vi "Netway Cal UI.vi"(11 "Calling VI Ref":refnum<vi>) -> ()   [LabVIEW 2013]
uses:
  Netway Driver/Type Defs/Communication Function Type Def.ctl
  <vilib>/Utility/miscctls.llb/LVRowAndColumnTypeDef.ctl
  <vilib>/Analysis/NI_AALPro.lvlib
  Type Defs/Target Cluster Type Def.ctl
  Type Defs/Setpoint Cluster Type Def.ctl
  Type Defs/Targets Type Def (Netway).ctl
  <vilib>/Utility/config.llb/NI_LVConfig.lvlib
  <userlib>/_OpenG.lib/array/array.llb/Remove Duplicates from 1D Array (DBL)__ogtk.vi
  Type Defs/Units Type Def (Netway).ctl
  Type Defs/Input or Output Type Def.ctl
  Type Defs/Channel Type Def (Netway).ctl
  <userlib>/_OpenG.lib/array/array.llb/Filter 1D Array (DBL)__ogtk.vi
panel:
  in  "Output Value Tab":enum32{"Page 1", "Page 2"}(tab)
  in  "OK Output":bool
  in  "Cancel Output":bool
  in  "Output Reading":dbl
  in  "Load Indicator Tab":enum32{"Page 1"}(tab)
  in  "Verify Tab":enum32{"Page 1", "Page 2"}(tab)
  in  "Hide Devs":bool
  in  "Auto":bool
  in  "Hide Cal Values":bool
  in  "Verify Edit":bool
  in  "Verify Table":string[][](table)=[["", "", "", "", ""], ["", "", "", "", ""], ["", "", "", "", ""], ["", "", "", "", ""], ["", "", "", "", ""], ["", "", "", "", ""], ["", "", "", "", ""], ["", "", "", "", ""], ["", "", "", "", ""], ["", "", "", "", ""]]
  in  "Verify Read":bool
  in  "ms":u32=1000
  in  "avg":i32=5
  in  "Header Tab":enum32{"Page 1", "Page 2"}(tab)
  in  "ZGW?":bool
  in  "Header OK":bool
  in  "Header Cancel":bool
  in  "Header Comments":string[][](table)=[["NETWAY80"], ["Software Revision:      8.11.B9            Firmware Revision:      8.12.B3            Flexray Revision:      8.12.B1"], [""]]
  in  "Cal Standards Table":string[][](table)=[["FLUKE DC CALIBRATOR", "1301"], ["AGILENT FUNCTION GENERATOR", "11401"], ["KEITHLEY MULTIMETER", "9570"], ["AGILENT SCOPEMETER", "11547"], ["", ""]]
  in  "Sys Cal Table":string[][](table)=[["", ""], ["", ""], ["", ""], ["", ""], ["", ""]]
  in  "Header Table 1":string[][](table)=[["11836"], ["SMART ENGINEERING (SET)"], ["NETWAY80"], ["4939"], ["NETWAY80 COMMS DAQ DEV"], ["SEE ATTACHED"], ["GOOD"], ["11357"]]
  in  "Header Table 2":string[][](table)=[["41409"], ["12"], ["41774"], ["CALIBRATION LAB"], ["22"], ["28"], ["KD"]]
  in  "App Dir":path
  in  "debug":bool=TRUE
  out "Row":i32
  in  "Main Tab":enum32{"Page 1", "Page 2"}(tab)
  in  "In/Out":T1
  in  "View Spreadsheet":bool
  in  "Header":bool
  out "Netway":i32 format="%04d"
  out "Cal Table":string[][](table)
  in  "Channel to Cal":T2=enum."AIO5"
  in  "Start Cal":bool
  in  "Confirm 1st Point":bool
  out "Reading Value 1":dbl caption="reading" format="%#.4g"
  in  "Cal Value 1":dbl caption="cal pt" format="%#.4g"
  in  "Confirm 2nd Point":bool
  out "Reading Value 2":dbl caption="reading" format="%#.4g"
  in  "Cal Value 2":dbl caption="cal pt" format="%#.4g"
  in  "Save Cal":bool
  out "f(x)":dbl caption="calibrated" format="%#.4g"
  out "a0":dbl format="%#.4g"
  out "a2":dbl format="%#.4g"
  in  "Cancel Cal":bool
  in  "Cal Unit":T3
  in  "Confirm 3rd Point":bool
  out "Reading Value 3":dbl caption="reading" format="%#.4g"
  in  "Cal Value 3":dbl caption="cal pt" format="%#.4g"
  out "a1":dbl format="%#.4g"
  in  "Start Verification":bool
  # "An external measurement device\nwas not detected.  Please manually\nenter value:"
  # "System Calibration Components"
  # "Calibration Standards Used"
  # "1)  Enter Header Info"
  # "2)  Select Channel to Calibrate"
  # "3) Start Procedure"
  # "- or -"
  # "4)  Take First Reading"
  # "5)  Take Second Reading"
  # "6)  Take Final Reading"
  # "7)  Review"
  # "8)  Confirm"
  # "Cal Spreadsheet"
  # "*Excel must be closed to return control to this app."
  # ","
  # ","
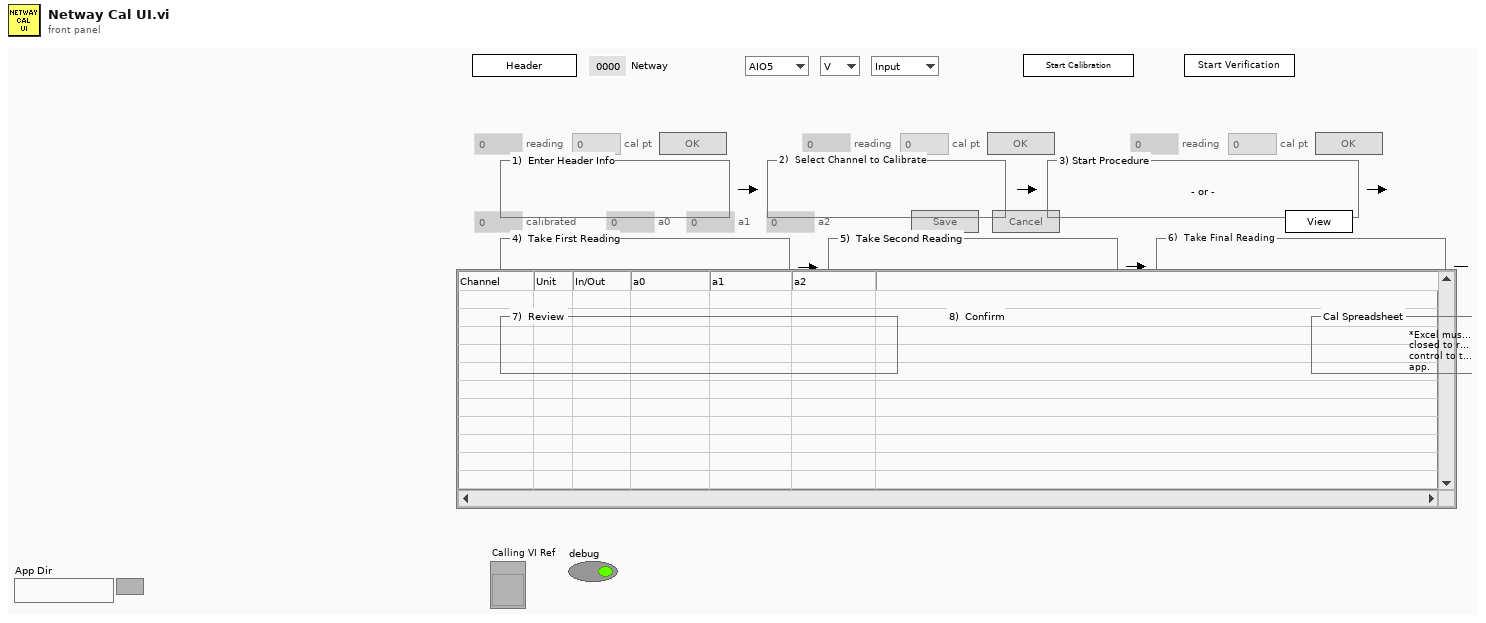
[diagram p1: front panel]
types:
  T1 = typedef "Input or Output Type Def.ctl" = enum16{"Input", "Output"}
  T2 = typedef "Channel Type Def (Netway).ctl" = enum16{"IO1", "IO2", "IO3", "IO4", "IO5", "IO6", "IO7", "IO8", "IO9", "IO10", "IO11", "IO12", "AIO1", "AIO2", "AIO3", "AIO4", "AIO5", "AIO6", "AIO7", "AIO8"}
  T3 = typedef "Units Type Def (Netway).ctl" = enum16{"V", "%", "Hz"}
  T4 = typedef "Targets Type Def (Netway).ctl" = cluster{"V0-11":T5, "V12-19":T5, "%":T5, "Hz":T5, "AO":T5, "%_out":T5, "Hz_out":T5, "AI0-11 Setpoints":T6, "AI12-19 Setpoints":T6, "Hz Setpoints":T6, "Duty Setpoints":T6}
  T5 = typedef "Target Cluster Type Def.ctl" = cluster{"target1":dbl, "target2":dbl, "target3":dbl, "target4":dbl, "target5":dbl, "target6":dbl, "target7":dbl, "target8":dbl, "target9":dbl, "target10":dbl}
  T6 = typedef "Setpoint Cluster Type Def.ctl" = cluster{"setpoint1":dbl, "setpoint2":dbl, "setpoint3":dbl}
  T7 = cluster{"Error":errorcluster, "Cal Log Header":string[], "Cal Files Base Path":path, "Cal Unit":T3, "Targets":T4, "Samples to Avg":i32, "Channel to Cal":T2, "Base Path":path, "Cal Targets Path":path, "Calling VI Ref":refnum<vi>, "Firmware Version":string, "debug":bool, "App Dir":path, "Verify Table":string[][], "Init Mean":bool, "Auto":bool, "Cal Template Path":path, "Netway":i32, "Cal Spreadsheet Path":path, "In/Out":T1, "Output Index":u8, "DMM Connected":bool, "Output Reading":bool, "Review":bool, "Verify Table Ref":refnum<vi>, "Verification":bool, "Init":bool, "Software Version":string, "ZGW Template Path":path, "ZGW?":bool}
  T8 = typedef "Communication Function Type Def.ctl" = enum16{"Find Devices", "Target Device"}
  T9 = enum8{"Enabled", "Disabled", "Disabled and Grayed Out"}
  T10 = typedef "LVRowAndColumnTypeDef.ctl" = cluster{"Row":i32, "Column":i32}
  T11 = enum32{"Bad", "Idle", "Run top level", "Running"}
  T12 = typedef "NI_LVConfig.lvlib/Config Data RefNum.ctl" = refnum<k1>
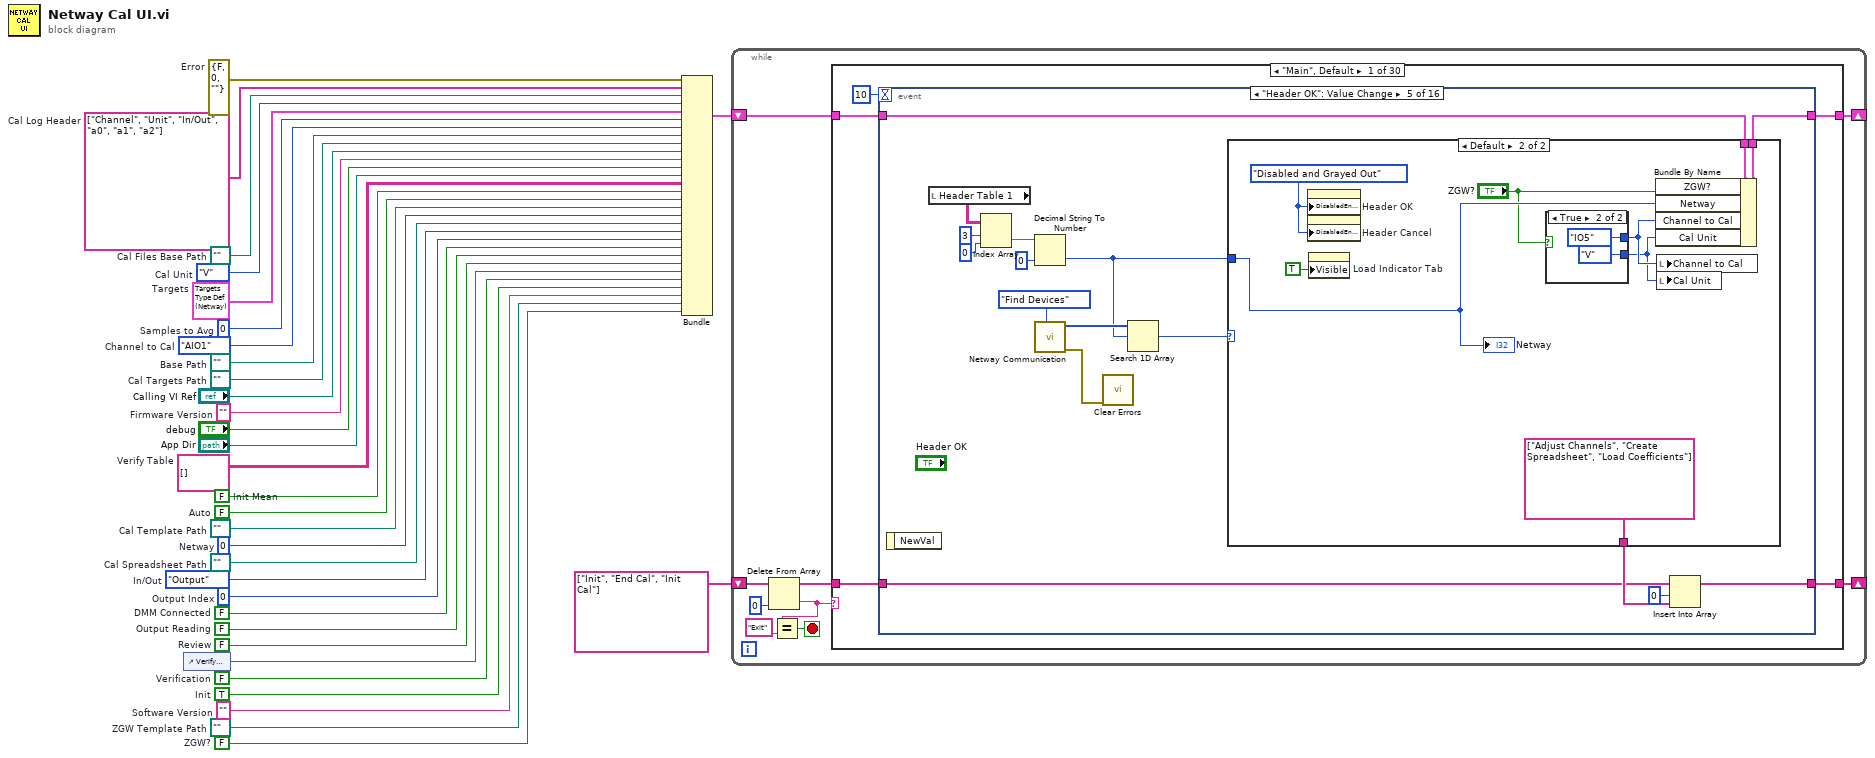
[diagram p0: block diagram]
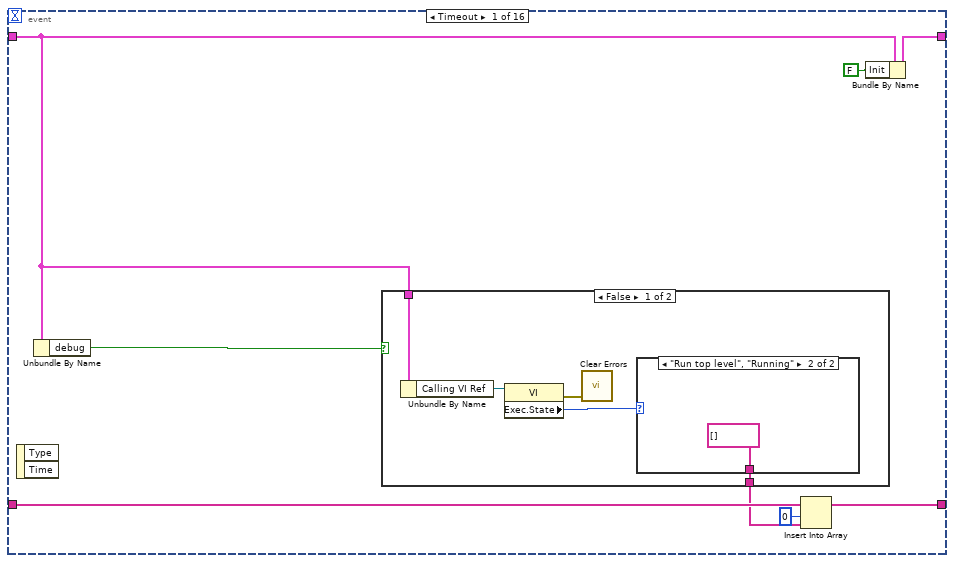
[diagram p2: hidden frame]
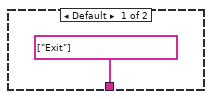
[diagram p3: hidden frame]
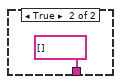
[diagram p4: hidden frame]
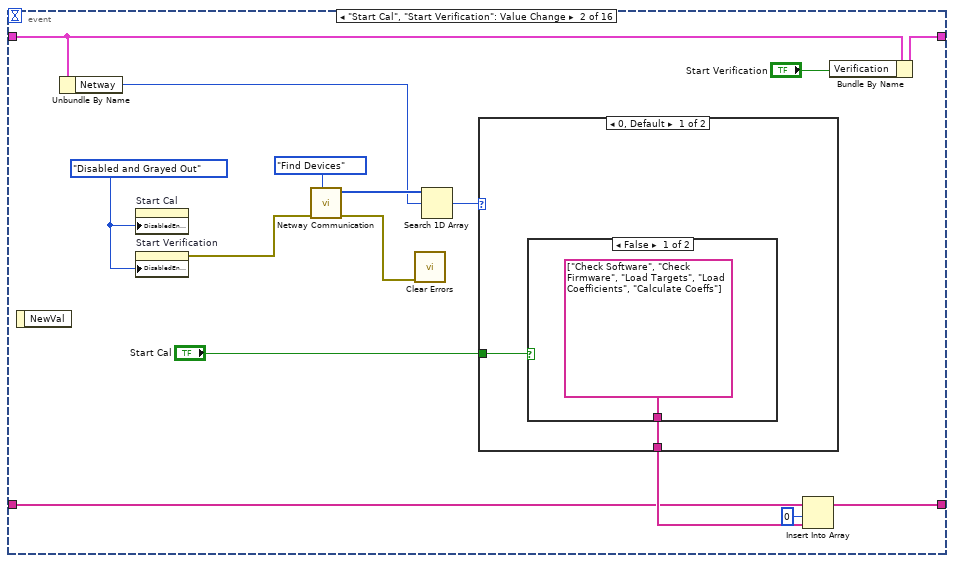
[diagram p5: hidden frame]
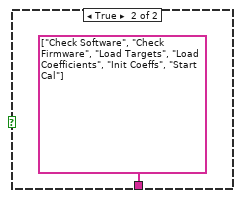
[diagram p6: hidden frame]
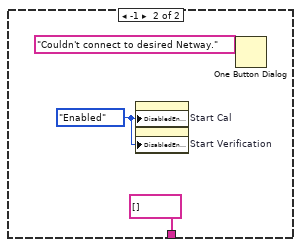
[diagram p7: hidden frame]
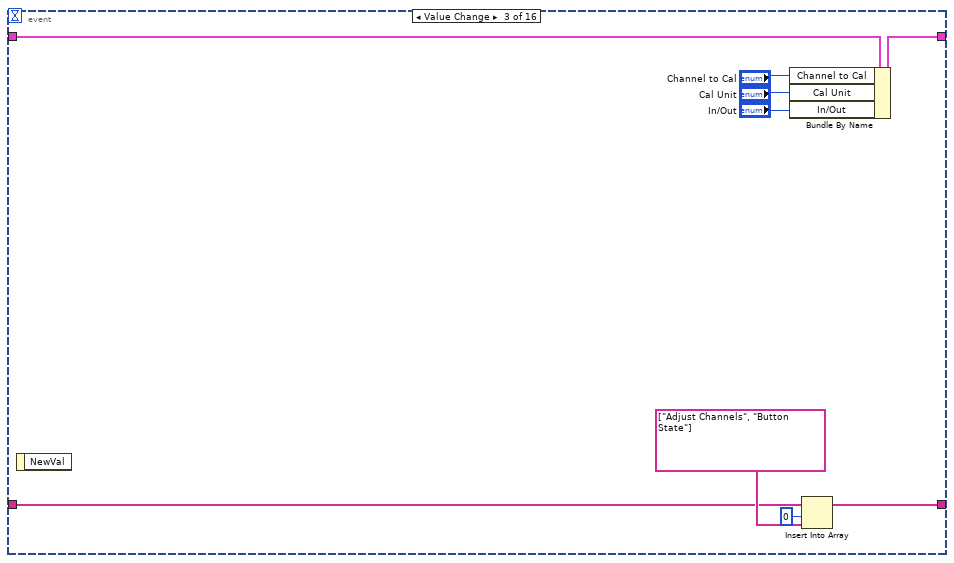
[diagram p8: hidden frame]
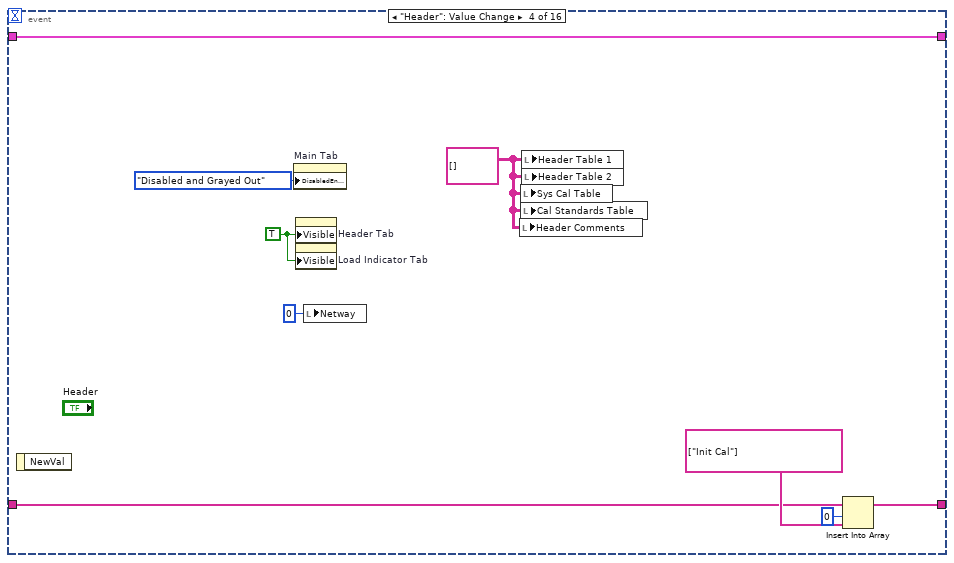
[diagram p9: hidden frame]
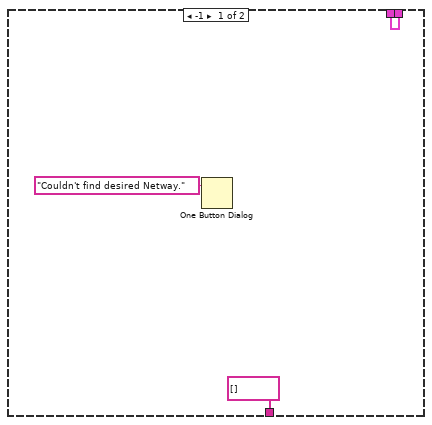
[diagram p10: hidden frame]
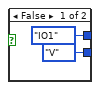
[diagram p11: hidden frame]
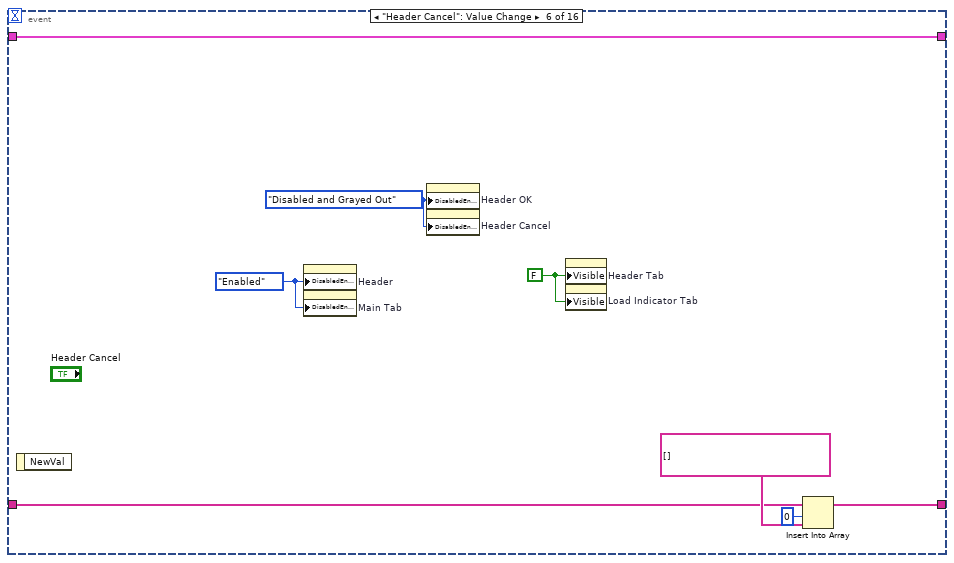
[diagram p12: hidden frame]
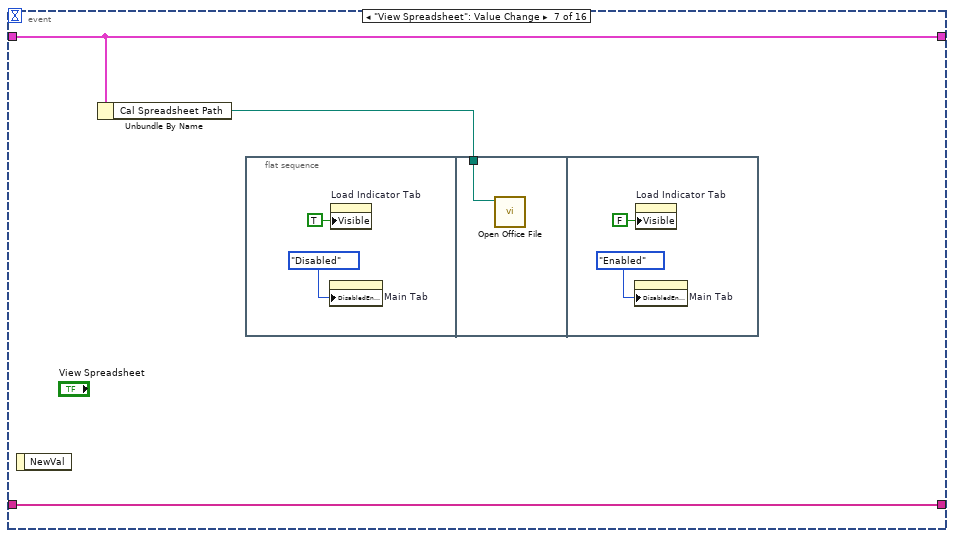
[diagram p13: hidden frame]
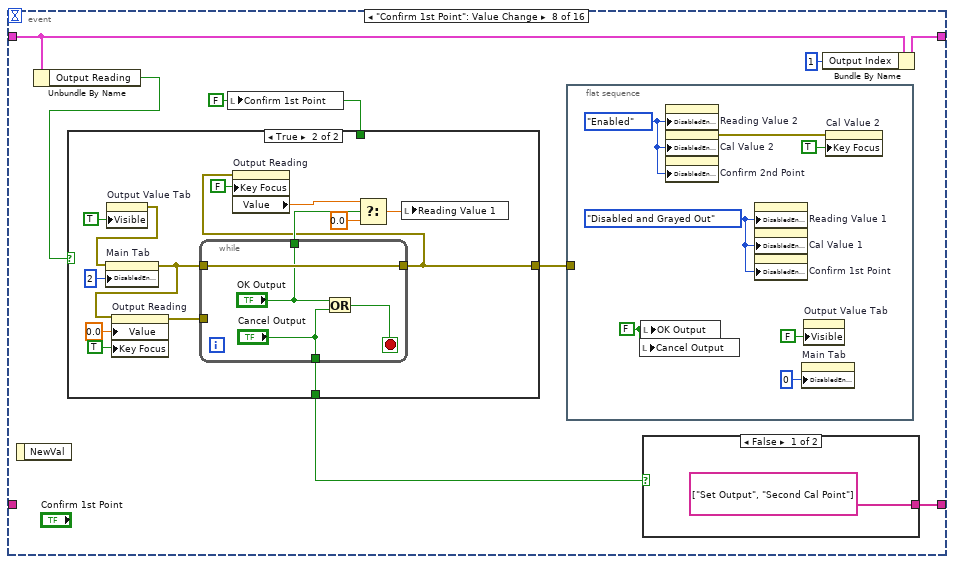
[diagram p14: hidden frame]
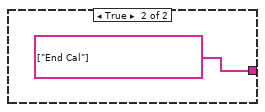
[diagram p15: hidden frame]
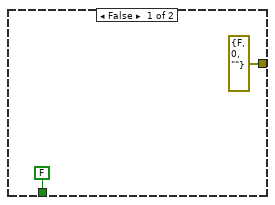
[diagram p16: hidden frame]
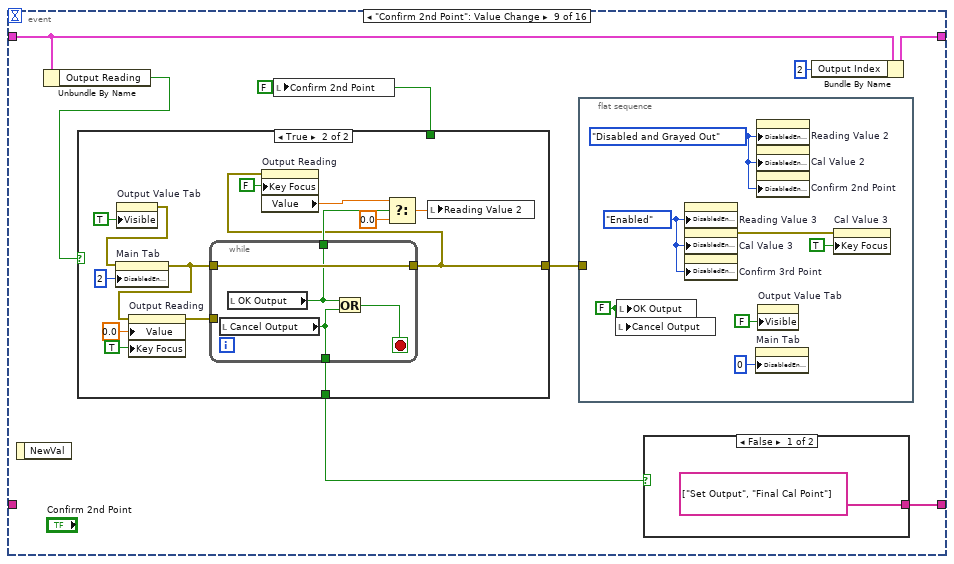
[diagram p17: hidden frame]
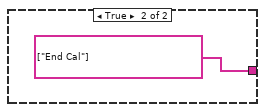
[diagram p18: hidden frame]
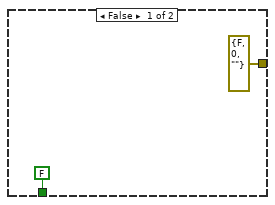
[diagram p19: hidden frame]
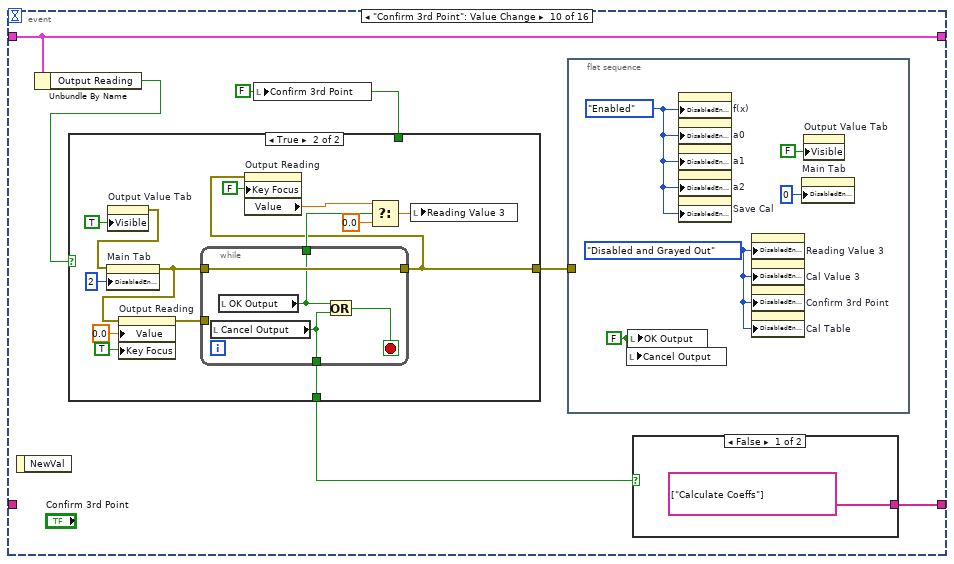
[diagram p20: hidden frame]
diagram:
  w1 = FALSE  # ZGW?
  w2 = path ""  # ZGW Template Path
  w3 = ""  # Software Version
  w4 = TRUE  # Init
  w5 = string[] ["Channel", "Unit", "In/Out", "a0", "a1", "a2"]  # Cal Log Header
  w6 = FALSE  # Verification
  w8 = FALSE  # Review
  w9 = FALSE  # Output Reading
  w10 = FALSE  # DMM Connected
  w11 = u8 0  # Output Index
  w12 = Channel_Type_Def_(Netway)."AIO1"  # Channel to Cal
  w13 = Input_or_Output_Type_Def."Output"  # In/Out
  w14 = Units_Type_Def_(Netway)."V"  # Cal Unit
  w15 = T4 {"V0-11"={"target1"=0.0, "target2"=0.0, "target3"=0.0, "target4"=0.0, "target5"=0.0, "target6"=0.0, "target7"=0.0, "target8"=0.0, "target9"=0.0, "target10"=0.0}, "V12-19"={"target1"=0.0, "target2"=0.0, "target3"=0.0, "target4"=0.0, "target5"=0.0, "target6"=0.0, "target7"=0.0, "target8"=0.0, "target9"=0.0, "target10"=0.0}, "%"={"target1"=0.0, "target2"=0.0, "target3"=0.0, "target4"=0.0, "target5"=0.0, "target6"=0.0, "target7"=0.0, "target8"=0.0, "target9"=0.0, "target10"=0.0}, "Hz"={"target1"=0.0, "target2"=0.0, "target3"=0.0, "target4"=0.0, "target5"=0.0, "target6"=0.0, "target7"=0.0, "target8"=0.0, "target9"=0.0, "target10"=0.0}, "AO"={"target1"=0.0, "target2"=0.0, "target3"=0.0, "target4"=0.0, "target5"=0.0, "target6"=0.0, "target7"=0.0, "target8"=0.0, "target9"=0.0, "target10"=0.0}, "%_out"={"target1"=0.0, "target2"=0.0, "target3"=0.0, "target4"=0.0, "target5"=0.0, "target6"=0.0, "target7"=0.0, "target8"=0.0, "target9"=0.0, "target10"=0.0}, "Hz_out"={"target1"=0.0, "target2"=0.0, "target3"=0.0, "target4"=0.0, "target5"=0.0, "target6"=0.0, "target7"=0.0, "target8"=0.0, "target9"=0.0, "target10"=0.0}, "AI0-11 Setpoints"={"setpoint1"=0.0, "setpoint2"=0.0, "setpoint3"=0.0}, "AI12-19 Setpoints"={"setpoint1"=0.0, "setpoint2"=0.0, "setpoint3"=0.0}, "Hz Setpoints"={"setpoint1"=0.0, "setpoint2"=0.0, "setpoint3"=0.0}, "Duty Setpoints"={"setpoint1"=0.0, "setpoint2"=0.0, "setpoint3"=0.0}}  # Targets
  w16 = path ""  # Cal Spreadsheet Path
  w17 = 0  # Netway
  w18 = path ""  # Cal Template Path
  w19 = FALSE  # Auto
  w20 = FALSE  # Init Mean
  w21 = string[][] []  # Verify Table
  w24 = ""  # Firmware Version
  w26 = path ""  # Cal Targets Path
  w27 = path ""  # Base Path
  w29 = 0  # Samples to Avg
  w30 = path ""  # Cal Files Base Path
  w28 = errorcluster {"status"=FALSE, "code"=0, "source"=""}  # Error
  n1 = control-ref of="Verify Table Ref"() -> (w7:refnum<vi>)
  n2 = Bundle("Error"=w28, "Cal Log Header"=w5, "Cal Files Base Path"=w30, "Cal Unit"=w14, "Targets"=w15, "Samples to Avg"=w29, "Channel to Cal"=w12, "Base Path"=w27, "Cal Targets Path"=w26, "Calling VI Ref"="Calling VI Ref", "Firmware Version"=w24, "debug"="debug", "App Dir"="App Dir", "Verify Table"=w21, "Init Mean"=w20, "Auto"=w19, "Cal Template Path"=w18, "Netway"=w17, "Cal Spreadsheet Path"=w16, "In/Out"=w13, "Output Index"=w11, "DMM Connected"=w10, "Output Reading"=w9, "Review"=w8, "Verify Table Ref"=w7, "Verification"=w6, "Init"=w4, "Software Version"=w3, "ZGW Template Path"=w2, "ZGW?"=w1) -> (w31:T7)  [unwired: 1 in]
  n3 = while {
    shift-right: [w38] -> _
    shift-left: string[] ["Init", "End Cal", "Init Cal"] -> [w41]
    shift-right: [w34] -> _
    shift-left: w31 -> [w35]
    stop <- w40 stop-if-true
    n4 = Delete From Array(array=w41, index=0) -> (deleted portion=w37:string, array with subset deleted=w39:string[])  [unwired: 1 in]
    n5 = Equal?(x=w37, y="Exit" ("x")) -> (x = y?=w40:bool)
    n6 = case shown="\"Main\", Default" w37 {
      tunnel: [w44 w391 w405 w412 w429 w578 w588 w591 w592 w623 w658 w683 w711 w777 w801 w830 w894 w909 w925 w967 w1024 w1051 w1087 w1100 w1129 string[] ["Recolor Tables", "Init Cal", "Button State"] w1149 w1161 w1175 w1189] -> w38
      tunnel: w39 -> [w45 w391 w405 w413 w429 w578 w588 w591 w593 w624 w659 w684 w711 w778 w800 w830 w893 w908 w924 w966 w1023 w1050 w1086 w1101 w1129 _ w1149 w1160 w1174 w1189]
      tunnel: w35 -> [w43 w385 w406 w420 w428 w579 w586 w590 w594 w625 w660 w682 w716 w783 w795 w829 w890 w901 w917 w949 w1015 w1047 w1089 w1102 w1130 w1138 w1151 w1159 w1173 w1188]
      tunnel: [w42 w394 w406 w419 w427 w579 w585 w590 w594 w622 w660 w682 w715 w783 w794 w829 w891 w900 w916 w948 w1021 w1047 w1088 w1102 w1130 w1138 w1150 w1159 w1173 w1188] -> w34
      frame "Main", Default {
        n7 = event shown="[4] \"Header OK\": Value Change" {
          selector: _ -> [_ _ _ _ _ _ _ _ _ _ _ _ _ _ _ _]
          dyn-events: _ -> [_ _ _ _ _ _ _ _ _ _ _ _ _ _ _ _]
          timeout: 10 -> [_ _ _ _ _ _ _ _ _ _ _ _ _ _ _ _]
          tunnel: [w54 w76 w88 w96 w114 w140 w143 w158 w193 w227 string[] ["Load Coefficients", "End Cal"] w270 w318 w348 w356 string[] ["Calc Dev", "Cal Review"]] -> w44
          tunnel: w45 -> [w53 w75 w89 w95 w113 w139 w143 _ _ _ _ w269 w318 w347 w356 _]
          tunnel: [w48 w69 w92 w97 w115 w138 w144 w153 w189 w229 w259 w266 w319 w351 w354 w362] -> w42
          tunnel: w43 -> [w49 w66 w93 w97 w116 w138 w144 w154 w190 w229 w259 w264 w319 w351 w355 w363]
          event Timeout {
            n8 = event-data() -> ()  [unwired: 1 in, 2 out]
            n9 = Unbundle By Name(w49) -> ("debug"=w51:bool)
            n10 = case shown="False" w51 {
              tunnel: [w59 string[] []] -> w52
              tunnel: w49 -> [w56 _]
              frame False {
                n11 = Unbundle By Name(w56) -> ("Calling VI Ref"=w58:refnum<vi>)
                n12 = property class="VI"(reference=w58) -> (error out=w55:errorcluster, "Exec.State"=w57:T11)  [unwired: 1 in, 1 out]
                n13 = call <vilib>:"Clear Errors.vi"("error in (no error)"=w55) -> ()  [unwired: 6 in, 1 out]
                n14 = case shown="\"Run top level\", \"Running\"" w57 {
                  tunnel: [string[] ["Exit"] string[] []] -> w59
                  frame Default {
                  }
                  frame "Run top level", "Running" {
                  }
                }
              }
              frame True {
              }
            }
            n15 = Insert Into Array(array=w53, index=0, new element=w52) -> (w54:string[])
            n16 = Bundle By Name(cluster=w49, "Init"=FALSE) -> (w48:T7)
          }
          event "Start Cal", "Start Verification": Value Change {
            w71 = T9."Disabled and Grayed Out" ("Disabled")
            n17 = event-data() -> ()  [unwired: 1 in, 1 out]
            n18 = Unbundle By Name(w66) -> ("Netway"=w64:i32)
            n19 = property on="Start Cal" class="Bool"("DisabledEnum"=w71) -> ()  [unwired: 2 in, 2 out]
            n20 = property on="Start Verification" class="Bool"("DisabledEnum"=w71) -> (error out=w65:errorcluster)  [unwired: 2 in, 1 out]
            n21 = call "Netway Communication.vi"("Function"=Communication_Function_Type_Def."Find Devices", "Error IN"=w65) -> ("Error OUT"=w72:errorcluster, "Serial Numbers"=w73:i32[])  [unwired: 6 in, 2 out]
            n22 = call <vilib>:"Clear Errors.vi"("error in (no error)"=w72) -> ()  [unwired: 6 in, 1 out]
            n23 = Search 1D Array(1D array=w73, element=w64) -> (index of element=w63:i32)  [unwired: 1 in]
            n24 = case shown="0, Default" w63 {
              tunnel: [w79 string[] []] -> w77
              tunnel: "Start Cal" -> [w78 _]
              frame 0, Default {
                n25 = case shown="False" w78 {
                  tunnel: [string[] ["Check Software", "Check Firmware", "Load Targets", "Load Coefficients", "Calculate Coeffs"] string[] ["Check Software", "Check Firmware", "Load Targets", "Load Coefficients", "Init Coeffs", "Start Cal"]] -> w79
                  frame False {
                  }
                  frame True {
                  }
                }
              }
              frame -1 {
                w82 = T9."Enabled" ("Disabled")
                n26 = property on="Start Cal" class="Bool"("DisabledEnum"=w82) -> ()  [unwired: 2 in, 2 out]
                n27 = property on="Start Verification" class="Bool"("DisabledEnum"=w82) -> ()  [unwired: 2 in, 2 out]
                n28 = One Button Dialog(message="Couldn't connect to desired Netway.") -> ()  [unwired: 1 in, 1 out]
              }
            }
            n29 = Insert Into Array(array=w75, index=0, new element=w77) -> (w76:string[])
            n30 = Bundle By Name(cluster=w66, "Verification"="Start Verification") -> (w69:T7)
          }
          event Value Change {
            n31 = event-data() -> ()  [unwired: 1 in, 1 out]
            n32 = Bundle By Name(cluster=w93, "Channel to Cal"="Channel to Cal", "Cal Unit"="Cal Unit", "In/Out"="In/Out") -> (w92:T7)
            n33 = Insert Into Array(array=w89, index=0, new element=string[] ["Adjust Channels", "Button State"]) -> (w88:string[])
          }
          event "Header": Value Change {
            w99 = string[][] [] ("Header Table 1")
            w100 = TRUE ("Visible")
            n34 = event-data() -> ()  [unwired: 1 in, 1 out]
            n35 = property on="Main Tab" class="TabCtl (strict)"("DisabledEnum"=T9."Disabled and Grayed Out" ("Disabled")) -> ()  [unwired: 2 in, 2 out]
            n36 = property on="Header Tab" class="TabCtl (strict)"("Visible"=w100) -> ()  [unwired: 2 in, 2 out]
            n37 = property on="Load Indicator Tab" class="TabCtl (strict)"("Visible"=w100) -> ()  [unwired: 2 in, 2 out]
            n38 = local write "Netway"(0 ("Netway")) -> ()
            n39 = local write "Header Comments"(w99) -> ()
            n40 = local write "Sys Cal Table"(w99) -> ()
            n41 = local write "Cal Standards Table"(w99) -> ()
            n42 = local write "Header Table 1"(w99) -> ()
            n43 = local write "Header Table 2"(w99) -> ()
            n44 = Insert Into Array(array=w95, index=0, new element=string[] ["Init Cal"]) -> (w96:string[])
          }
          event "Header OK": Value Change {
            n45 = event-data() -> ()  [unwired: 1 in, 1 out]
            n46 = local read "Header Table 1"() -> (w111:string[][])
            n47 = Index Array(array=w111, index (row)=3, index (col)=0 ("disabled index (col)")) -> (element=w108:string)
            n48 = Decimal String To Number(string=w108, default (0L)=0 ("DAQ Rack")) -> (number=w105:i32)  [unwired: 1 in, 1 out]
            n49 = call "Netway Communication.vi"("Function"=Communication_Function_Type_Def."Find Devices") -> ("Error OUT"=w104:errorcluster, "Serial Numbers"=w106:i32[])  [unwired: 7 in, 2 out]
            n50 = call <vilib>:"Clear Errors.vi"("error in (no error)"=w104) -> ()  [unwired: 6 in, 1 out]
            n51 = Search 1D Array(1D array=w106, element=w105) -> (index of element=w103:i32)  [unwired: 1 in]
            n52 = case shown="Default" w103 {
              tunnel: [string[] [] string[] ["Adjust Channels", "Create Spreadsheet", "Load Coefficients"]] -> w117
              tunnel: w116 -> [w121 w128]
              tunnel: [w121 w127] -> w115
              tunnel: w105 -> [_ w124]
              frame -1 {
                n53 = One Button Dialog(message="Couldn't find desired Netway.") -> ()  [unwired: 1 in, 1 out]
              }
              frame Default {
                w129 = T9."Disabled and Grayed Out" ("Disabled")
                n54 = property on="Header OK" class="Bool"("DisabledEnum"=w129) -> ()  [unwired: 2 in, 2 out]
                n55 = property on="Header Cancel" class="Bool"("DisabledEnum"=w129) -> ()  [unwired: 2 in, 2 out]
                n56 = property on="Load Indicator Tab" class="TabCtl (strict)"("Visible"=TRUE) -> ()  [unwired: 2 in, 2 out]
                n57 = case shown="True" "ZGW?" {
                  tunnel: [Channel_Type_Def_(Netway)."IO1" ("Channel to Cal") Channel_Type_Def_(Netway)."IO5" ("Channel to Cal")] -> w126
                  tunnel: [Units_Type_Def_(Netway)."V" ("Cal Unit") Units_Type_Def_(Netway)."V" ("Cal Unit")] -> w125
                  frame False {
                  }
                  frame True {
                  }
                }
                n58 = Bundle By Name(cluster=w128, "ZGW?"="ZGW?", "Netway"=w124, "Channel to Cal"=w126, "Cal Unit"=w125) -> (w127:T7)
                n59 = local write "Channel to Cal"(w126) -> ()
                n60 = local write "Cal Unit"(w125) -> ()
                "Netway" <- w124
              }
            }
            n61 = Insert Into Array(array=w113, index=0, new element=w117) -> (w114:string[])
          }
          event "Header Cancel": Value Change {
            w136 = FALSE ("Visible")
            w135 = T9."Enabled" ("Disabled")
            w137 = T9."Disabled and Grayed Out" ("Disabled")
            n62 = event-data() -> ()  [unwired: 1 in, 1 out]
            n63 = property on="Header" class="Bool"("DisabledEnum"=w135) -> ()  [unwired: 2 in, 2 out]
            n64 = property on="Main Tab" class="TabCtl (strict)"("DisabledEnum"=w135) -> ()  [unwired: 2 in, 2 out]
            n65 = property on="Header OK" class="Bool"("DisabledEnum"=w137) -> ()  [unwired: 2 in, 2 out]
            n66 = property on="Header Cancel" class="Bool"("DisabledEnum"=w137) -> ()  [unwired: 2 in, 2 out]
            n67 = property on="Header Tab" class="TabCtl (strict)"("Visible"=w136) -> ()  [unwired: 2 in, 2 out]
            n68 = property on="Load Indicator Tab" class="TabCtl (strict)"("Visible"=w136) -> ()  [unwired: 2 in, 2 out]
            n69 = Insert Into Array(array=w139, index=0, new element=string[] []) -> (w140:string[])
          }
          event "View Spreadsheet": Value Change {
            n70 = event-data() -> ()  [unwired: 1 in, 1 out]
            n71 = Unbundle By Name(w144) -> ("Cal Spreadsheet Path"=w145:path)
            n72 = flat-sequence {
              tunnel: w145 -> [w148]
              frame #0 {
                n73 = property on="Main Tab" class="TabCtl (strict)"("DisabledEnum"=T9."Disabled" ("Disabled")) -> ()  [unwired: 2 in, 2 out]
                n74 = property on="Load Indicator Tab" class="TabCtl (strict)"("Visible"=TRUE) -> ()  [unwired: 2 in, 2 out]
              }
              frame #1 {
                n75 = call "Open Office File.vi"("Selection a Word (.doc, .docx), Excel (.xls, .xlsx), or Powerpoint (.ppt, .pptx) Document..."=w148) -> ()  [unwired: 10 in, 1 out]
              }
              frame #2 {
                n76 = property on="Main Tab" class="TabCtl (strict)"("DisabledEnum"=T9."Enabled" ("Disabled")) -> ()  [unwired: 2 in, 2 out]
                n77 = property on="Load Indicator Tab" class="TabCtl (strict)"("Visible"=FALSE) -> ()  [unwired: 2 in, 2 out]
              }
            }
          }
          event "Confirm 1st Point": Value Change {
            w151 = FALSE ("Confirm 1st Point")
            n78 = event-data() -> ()  [unwired: 1 in, 1 out]
            n79 = Unbundle By Name(w154) -> ("Output Reading"=w156:bool)
            n80 = case shown="True" w156 {
              tunnel: [errorcluster {"status"=FALSE, "code"=0, "source"=""} ("error out") w163] -> w157
              tunnel: [FALSE ("Cancel Output") w173] -> w155
              tunnel: w151 -> [_ _]
              frame False {
              }
              frame True {
                n81 = property on="Output Value Tab" class="TabCtl (strict)"("Visible"=TRUE) -> (error out=w174:errorcluster)  [unwired: 2 in, 1 out]
                n82 = property on="Main Tab" class="TabCtl (strict)"(error in=w174, "DisabledEnum"=2) -> (error out=w169:errorcluster)  [unwired: 1 in, 1 out]
                n83 = property on="Output Reading" class="DigNum (strict)"(error in=w169, "Value"=0.0 ("Output Reading"), "Key Focus"=TRUE) -> (error out=w170:errorcluster)  [unwired: 1 in, 1 out]
                n84 = while {
                  tunnel: [w179] -> w163
                  tunnel: w169 -> [w179]
                  tunnel: ["Cancel Output"] -> w173
                  tunnel: w170 -> [_]
                  tunnel: ["OK Output"] -> w165
                  stop <- w180 stop-if-true
                  n85 = Or(x="OK Output", y="Cancel Output") -> (x .or. y?=w180:bool)
                }
                n86 = property on="Output Reading" class="DigNum (strict)"(error in=w163, "Key Focus"=FALSE) -> ("Value"=w167:dbl)  [unwired: 1 in, 2 out]
                n87 = Select(t=w167, s=w165, f=0.0) -> (s? t:f=w164:dbl)
                n88 = local write "Reading Value 1"(w164) -> ()
              }
            }
            n89 = local write "Confirm 1st Point"(w151) -> ()
            n90 = flat-sequence {
              tunnel: w157 -> [_]
              frame #0 {
                w181 = FALSE ("OK Output")
                w185 = T9."Disabled and Grayed Out" ("Disabled")
                w186 = T9."Enabled" ("Disabled")
                n91 = local write "Cancel Output"(w181) -> ()
                n92 = local write "OK Output"(w181) -> ()
                n93 = property on="Reading Value 2" class="DigNum (strict)"("DisabledEnum"=w186) -> ()  [unwired: 2 in, 2 out]
                n94 = property on="Cal Value 2" class="DigNum (strict)"("DisabledEnum"=w186) -> (error out=w184:errorcluster)  [unwired: 2 in, 1 out]
                n95 = property on="Confirm 2nd Point" class="Bool (strict)"("DisabledEnum"=w186) -> ()  [unwired: 2 in, 2 out]
                n96 = property on="Reading Value 1" class="DigNum (strict)"("DisabledEnum"=w185) -> ()  [unwired: 2 in, 2 out]
                n97 = property on="Cal Value 1" class="DigNum (strict)"("DisabledEnum"=w185) -> ()  [unwired: 2 in, 2 out]
                n98 = property on="Confirm 1st Point" class="Bool (strict)"("DisabledEnum"=w185) -> ()  [unwired: 2 in, 2 out]
                n99 = property on="Main Tab" class="TabCtl (strict)"("DisabledEnum"=0) -> ()  [unwired: 2 in, 2 out]
                n100 = property on="Output Value Tab" class="TabCtl (strict)"("Visible"=FALSE) -> ()  [unwired: 2 in, 2 out]
                n101 = property on="Cal Value 2" class="DigNum (strict)"(error in=w184, "Key Focus"=TRUE) -> ()  [unwired: 1 in, 2 out]
              }
            }
            n102 = case shown="False" w155 {
              tunnel: [string[] ["Set Output", "Second Cal Point"] string[] ["End Cal"]] -> w158
              frame False {
              }
              frame True {
              }
            }
            n103 = Bundle By Name(cluster=w154, "Output Index"=u8 1) -> (w153:T7)
          }
          event "Confirm 2nd Point": Value Change {
            w188 = FALSE ("Confirm 1st Point")
            n104 = event-data() -> ()  [unwired: 1 in, 1 out]
            n105 = Unbundle By Name(w190) -> ("Output Reading"=w195:bool)
            n106 = case shown="True" w195 {
              tunnel: [errorcluster {"status"=FALSE, "code"=0, "source"=""} ("error out") w200] -> w194
              tunnel: [FALSE ("Cancel Output") w210] -> w192
              tunnel: w188 -> [_ _]
              frame False {
              }
              frame True {
                n107 = property on="Output Value Tab" class="TabCtl (strict)"("Visible"=TRUE) -> (error out=w211:errorcluster)  [unwired: 2 in, 1 out]
                n108 = property on="Main Tab" class="TabCtl (strict)"(error in=w211, "DisabledEnum"=2) -> (error out=w206:errorcluster)  [unwired: 1 in, 1 out]
                n109 = property on="Output Reading" class="DigNum (strict)"(error in=w206, "Value"=0.0 ("Output Reading"), "Key Focus"=TRUE) -> (error out=w207:errorcluster)  [unwired: 1 in, 1 out]
                n110 = while {
                  tunnel: [w216] -> w200
                  tunnel: w206 -> [w216]
                  tunnel: [w215] -> w210
                  tunnel: w207 -> [_]
                  tunnel: [w214] -> w202
                  stop <- w217 stop-if-true
                  n111 = local read "Cancel Output"() -> (w215:bool)
                  n112 = local read "OK Output"() -> (w214:bool)
                  n113 = Or(x=w214, y=w215) -> (x .or. y?=w217:bool)
                }
                n114 = property on="Output Reading" class="DigNum (strict)"(error in=w200, "Key Focus"=FALSE) -> ("Value"=w204:dbl)  [unwired: 1 in, 2 out]
                n115 = Select(t=w204, s=w202, f=0.0) -> (s? t:f=w201:dbl)
                n116 = local write "Reading Value 2"(w201) -> ()
              }
            }
            n117 = local write "Confirm 2nd Point"(w188) -> ()
            n118 = flat-sequence {
              tunnel: w194 -> [_]
              frame #0 {
                w218 = FALSE ("OK Output")
                w223 = T9."Enabled" ("Disabled")
                w224 = T9."Disabled and Grayed Out" ("Disabled")
                n119 = local write "Cancel Output"(w218) -> ()
                n120 = local write "OK Output"(w218) -> ()
                n121 = property on="Reading Value 3" class="DigNum (strict)"("DisabledEnum"=w223) -> ()  [unwired: 2 in, 2 out]
                n122 = property on="Cal Value 3" class="DigNum (strict)"("DisabledEnum"=w223) -> (error out=w221:errorcluster)  [unwired: 2 in, 1 out]
                n123 = property on="Confirm 3rd Point" class="Bool (strict)"("DisabledEnum"=w223) -> ()  [unwired: 2 in, 2 out]
                n124 = property on="Main Tab" class="TabCtl (strict)"("DisabledEnum"=0) -> ()  [unwired: 2 in, 2 out]
                n125 = property on="Reading Value 2" class="DigNum (strict)"("DisabledEnum"=w224) -> ()  [unwired: 2 in, 2 out]
                n126 = property on="Cal Value 2" class="DigNum (strict)"("DisabledEnum"=w224) -> ()  [unwired: 2 in, 2 out]
                n127 = property on="Confirm 2nd Point" class="Bool (strict)"("DisabledEnum"=w224) -> ()  [unwired: 2 in, 2 out]
                n128 = property on="Output Value Tab" class="TabCtl (strict)"("Visible"=FALSE) -> ()  [unwired: 2 in, 2 out]
                n129 = property on="Cal Value 3" class="DigNum (strict)"(error in=w221, "Key Focus"=TRUE) -> ()  [unwired: 1 in, 2 out]
              }
            }
            n130 = case shown="False" w192 {
              tunnel: [string[] ["Set Output", "Final Cal Point"] string[] ["End Cal"]] -> w193
              frame False {
              }
              frame True {
              }
            }
            n131 = Bundle By Name(cluster=w190, "Output Index"=u8 2) -> (w189:T7)
          }
          event "Confirm 3rd Point": Value Change {
            w225 = FALSE ("Confirm 1st Point")
            n132 = event-data() -> ()  [unwired: 1 in, 1 out]
            n133 = Unbundle By Name(w229) -> ("Output Reading"=w230:bool)
            n134 = case shown="True" w230 {
              tunnel: [errorcluster {"status"=FALSE, "code"=0, "source"=""} ("error out") w235] -> w228
              tunnel: [FALSE ("Cancel Output") w245] -> w226
              tunnel: w225 -> [_ _]
              frame False {
              }
              frame True {
                n135 = property on="Output Value Tab" class="TabCtl (strict)"("Visible"=TRUE) -> (error out=w246:errorcluster)  [unwired: 2 in, 1 out]
                n136 = property on="Main Tab" class="TabCtl (strict)"(error in=w246, "DisabledEnum"=2) -> (error out=w241:errorcluster)  [unwired: 1 in, 1 out]
                n137 = property on="Output Reading" class="DigNum (strict)"(error in=w241, "Value"=0.0 ("Output Reading"), "Key Focus"=TRUE) -> (error out=w242:errorcluster)  [unwired: 1 in, 1 out]
                n138 = while {
                  tunnel: [w251] -> w235
                  tunnel: w241 -> [w251]
                  tunnel: [w250] -> w245
                  tunnel: w242 -> [_]
                  tunnel: [w249] -> w237
                  stop <- w252 stop-if-true
                  n139 = local read "Cancel Output"() -> (w250:bool)
                  n140 = local read "OK Output"() -> (w249:bool)
                  n141 = Or(x=w249, y=w250) -> (x .or. y?=w252:bool)
                }
                n142 = property on="Output Reading" class="DigNum (strict)"(error in=w235, "Key Focus"=FALSE) -> ("Value"=w239:dbl)  [unwired: 1 in, 2 out]
                n143 = Select(t=w239, s=w237, f=0.0) -> (s? t:f=w236:dbl)
                n144 = local write "Reading Value 3"(w236) -> ()
              }
            }
            n145 = local write "Confirm 3rd Point"(w225) -> ()
            n146 = flat-sequence {
              tunnel: w228 -> [_]
              frame #0 {
                w253 = FALSE ("OK Output")
                w256 = T9."Enabled" ("Disabled")
                w257 = T9."Disabled and Grayed Out" ("Disabled")
                n147 = local write "Cancel Output"(w253) -> ()
                n148 = local write "OK Output"(w253) -> ()
                n149 = property on="f(x)" class="DigNum (strict)"("DisabledEnum"=w256) -> ()  [unwired: 2 in, 2 out]
                n150 = property on="a0" class="DigNum (strict)"("DisabledEnum"=w256) -> ()  [unwired: 2 in, 2 out]
                n151 = property on="a1" class="DigNum (strict)"("DisabledEnum"=w256) -> ()  [unwired: 2 in, 2 out]
                n152 = property on="a2" class="DigNum (strict)"("DisabledEnum"=w256) -> ()  [unwired: 2 in, 2 out]
                n153 = property on="Save Cal" class="Bool"("DisabledEnum"=w256) -> ()  [unwired: 2 in, 2 out]
                n154 = property on="Reading Value 3" class="DigNum (strict)"("DisabledEnum"=w257) -> ()  [unwired: 2 in, 2 out]
                n155 = property on="Cal Value 3" class="DigNum (strict)"("DisabledEnum"=w257) -> ()  [unwired: 2 in, 2 out]
                n156 = property on="Confirm 3rd Point" class="Bool (strict)"("DisabledEnum"=w257) -> ()  [unwired: 2 in, 2 out]
                n157 = property on="Cal Table" class="Tbl (strict)"("DisabledEnum"=w257) -> ()  [unwired: 2 in, 2 out]
                n158 = property on="Main Tab" class="TabCtl (strict)"("DisabledEnum"=0) -> ()  [unwired: 2 in, 2 out]
                n159 = property on="Output Value Tab" class="TabCtl (strict)"("Visible"=FALSE) -> ()  [unwired: 2 in, 2 out]
              }
            }
            n160 = case shown="False" w226 {
              tunnel: [string[] ["Calculate Coeffs"] string[] ["End Cal"]] -> w227
              frame False {
              }
              frame True {
              }
            }
          }
          event "Cancel Cal": Value Change {
            n161 = event-data() -> ()  [unwired: 1 in, 1 out]
          }
          event "Verify Read": Value Change {
            n162 = event-data() -> ()  [unwired: 1 in, 1 out]
            n163 = Unbundle By Name(w264) -> ("Output Index"=w262:u8, "Output Reading"=w263:bool)
            n164 = case shown="True" "Verify Read" {
              tunnel: [FALSE ("Verify Read") FALSE ("Verify Read")] -> w260
              tunnel: [w273 w275] -> w270
              tunnel: w269 -> [w273 _]
              tunnel: w264 -> [w272 w284]
              tunnel: [w272 w283] -> w267
              tunnel: w263 -> [_ w279]
              tunnel: w262 -> [w271 w277]
              tunnel: [w271 w276] -> w261
              frame False {
              }
              frame True {
                n165 = case shown="True" w279 {
                  tunnel: [w293 w294] -> w278
                  tunnel: [string[] ["Calc Dev", "Set Output", "Cal Review"] w304] -> w275
                  frame False {
                    n166 = local read "f(x)"() -> (w293:dbl)
                  }
                  frame True {
                    n167 = property on="Output Value Tab" class="TabCtl (strict)"("Visible"=TRUE) -> (error out=w309:errorcluster)  [unwired: 2 in, 1 out]
                    n168 = property on="Main Tab" class="TabCtl (strict)"(error in=w309, "DisabledEnum"=2) -> (error out=w300:errorcluster)  [unwired: 1 in, 1 out]
                    n169 = property on="Output Reading" class="DigNum (strict)"(error in=w300, "Value"=0.0 ("Output Reading"), "Key Focus"=TRUE) -> (error out=w301:errorcluster)  [unwired: 1 in, 1 out]
                    n170 = while {
                      tunnel: [w316] -> w295
                      tunnel: w300 -> [w316]
                      tunnel: [w315] -> w305
                      tunnel: w301 -> [_]
                      tunnel: [w314] -> w296
                      stop <- w317 stop-if-true
                      n171 = local read "Cancel Output"() -> (w315:bool)
                      n172 = local read "OK Output"() -> (w314:bool)
                      n173 = Or(x=w314, y=w315) -> (x .or. y?=w317:bool)
                    }
                    n174 = property on="Output Reading" class="DigNum (strict)"(error in=w295, "Key Focus"=FALSE) -> ("Value"=w298:dbl)  [unwired: 1 in, 2 out]
                    n175 = case shown="False" w305 {
                      tunnel: [string[] ["Calc Dev", "Set Output", "Cal Review"] string[] ["End Cal"]] -> w304
                      frame False {
                      }
                      frame True {
                      }
                    }
                    n176 = Select(t=w298, s=w296, f=0.0) -> (s? t:f=w294:dbl)
                    n177 = property on="Output Value Tab" class="TabCtl (strict)"(error in=w295, "Visible"=FALSE) -> (error out=w308:errorcluster)  [unwired: 1 in, 1 out]
                    n178 = property on="Main Tab" class="TabCtl (strict)"(error in=w308, "DisabledEnum"=0) -> ()  [unwired: 1 in, 2 out]
                  }
                }
                n179 = Increment(x=w277) -> (x+1=w276:u8)
                n180 = local read "Verify Table"() -> (w285:string[][])
                n181 = local read "Row"() -> (w288:i32)
                n182 = Number To Fractional String(number=w278) -> (F-format string=w287:string)  [unwired: 3 in]
                n183 = Replace Array Subset(array=w285, new element=w287, index (row)=w288, index (col)=1 ("disabled index (col)")) -> (w280:string[][])
                n184 = Increment(x=w288) -> (x+1=w290:i32)
                n185 = Bundle(w290, "disabled index (col)"=1) -> (w281:cluster{i32, "disabled index (col)":i32})  [unwired: 1 in]
                n186 = Bundle By Name(cluster=w284, "Verify Table"=w280) -> (w283:T7)
                n187 = property on="Verify Table" class="Tbl (strict)"("Key Focus"=TRUE, "EditPos"=w281, "Value"=w280) -> ()  [unwired: 2 in, 2 out]
              }
            }
            n188 = local write "Cancel Output"(w260) -> ()
            n189 = local write "OK Output"(w260) -> ()
            n190 = local write "Verify Read"(w260) -> ()
            n191 = Bundle By Name(cluster=w267, "Init Mean"=TRUE ("initialize"), "Output Index"=w261) -> (w266:T7)
          }
          event "Verify Edit": Value Change {
            n192 = event-data() -> ()  [unwired: 1 in, 1 out]
            n193 = disable-structure shown="Disabled" {
              disable-tunnel: w319 -> [w321 _]
              frame Disabled {
                n194 = case shown="False" "Verify Edit" {
                  tunnel: w321 -> [w323 _]
                  frame False {
                    w327 = T9."Enabled" ("Disabled")
                    w338 = TRUE ("Visible")
                    n195 = Unbundle By Name(w323) -> ("Cal Targets Path"=w322:path)
                    n196 = local read "Cal Unit"() -> (w333:T3)
                    n197 = property on="Cal Unit" class="Enum (strict)"() -> ("Strings []"=w332:string[])  [unwired: 2 in, 2 out]
                    n198 = local read "Channel to Cal"() -> (w324:T2)
                    n199 = Index Array(array=w332, index=w333) -> (element=w326:string)
                    n200 = case shown="\"V\"" w326 {
                      selector: w326 -> [w339 _]
                      tunnel: [w339 w340] -> w325
                      tunnel: w324 -> [_ w341]
                      frame "False", Default {
                      }
                      frame "V" {
                        n201 = case shown="\"AIO1\"..\"AIO8\"" w341 {
                          tunnel: ["V0-11" "V12-19"] -> w340
                          frame "IO1".."IO12", Default {
                          }
                          frame "AIO1".."AIO8" {
                          }
                        }
                      }
                    }
                    n202 = Index Array(array=w336, index (col)=2 ("disabled index (col)")) -> (element=w329)  [unwired: 1 in]
                    n203 = Build Array(string[] ["target1", "target2", "target3", "target4", "target5", "target6", "target7", "target8", "target9", "target10"], w329) -> (w331:string[][])
                    n204 = Replace Array Subset(new element=w329, index (col)=1 ("disabled index (col)")) -> (array=w336:void[], w337:void[])  [unwired: 1 in]
                    n205 = Transpose 2D Array(2D array=w331) -> (transposed array=w330:string[][])
                    n206 = call "String Array to INI.vi"("Path"=w322, "Section"=w325, "Array"=w330) -> ()  [unwired: 12 in, 1 out]
                  }
                  frame True {
                    w344 = T9."Disabled and Grayed Out" ("Disabled")
                    w345 = FALSE ("Visible")
                  }
                }
              }
              frame Enabled {
              }
            }
          }
          event "Save Cal": Value Change {
            n207 = event-data() -> ()  [unwired: 1 in, 1 out]
            n208 = property on="Cal Table" class="Tbl (strict)"("DisabledEnum"=T9."Enabled" ("Disabled")) -> ()  [unwired: 2 in, 2 out]
            n209 = property on="Verify Tab" class="TabCtl (strict)"("Visible"=FALSE) -> ()  [unwired: 2 in, 2 out]
            n210 = Insert Into Array(array=w347, index=0, new element=string[] ["Save Cal"]) -> (w348:string[])
          }
          event "Auto": Value Change {
            n211 = event-data() -> ()  [unwired: 1 in, 1 out]
            n212 = case shown="True" "Auto" {
              frame False {
              }
              frame True {
                n213 = local read "Row"() -> (w360:i32)
                n214 = Bundle("Row"=w360, "disabled index (col)"=1) -> (w358:cluster{"Row":i32, "disabled index (col)":i32})  [unwired: 1 in]
                n215 = property on="Verify Table" class="Tbl (strict)"("Key Focus"=TRUE, "EditPos"=w358) -> ()  [unwired: 2 in, 2 out]
              }
            }
            n216 = Bundle By Name(cluster=w355, "Auto"="Auto") -> (w354:T7)
          }
          event "Verify Table": Value Change {
            n217 = event-data() -> ()  [unwired: 1 in, 1 out]
            n218 = Bundle By Name(cluster=w363, "Verify Table"="Verify Table") -> (w362:T7)
          }
        }
      }
      frame "Init" {
        w370 = FALSE ("OK Output")
        n219 = Unbundle By Name(w385) -> ("debug"=w377:bool, "App Dir"=w378:path)
        n220 = property on="Output Value Tab" class="TabCtl (strict)"("Visible"=FALSE) -> ()  [unwired: 2 in, 2 out]
        n221 = property on="Cal Table" class="Tbl (strict)"("Active Cell"=T10 {"Row"=-2, "Column"=-2} ("Active Cell:Active Cell"), "Cell BG Color"=u32 16448250) -> ()  [unwired: 2 in, 2 out]
        n222 = Select(t=path "C:/Documents and Settings/tzt79f/My Documents/Projects/Calibration Utility/Source", s=w377, f=w378) -> (s? t:f=w375:path)
        n223 = Build Path(base path=w375, name or relative path="App Config.ini") -> (appended path=w386:path)
        n224 = Build Path(base path=w375, name or relative path="Calibration UIs\\Netway") -> (appended path=w382:path)
        n225 = call "Read App Config.vi"("App Config Path"=w386) -> ("Cal Files Path"=w390:path)  [unwired: 9 in, 1 out]
        n226 = Build Path(base path=w390, name or relative path="Netway") -> (appended path=w381:path)
        n227 = Build Path(base path=w382, name or relative path="Cal Targets.ini") -> (appended path=w383:path)
        n228 = Create Folder(path (use dialog)=w381) -> (error out=w392:errorcluster)  [unwired: 2 in, 2 out]
        n229 = call <vilib>:"Clear Errors.vi"("error in (no error)"=w392) -> ("error out"=w380:errorcluster)  [unwired: 6 in]
        n230 = for {
          tunnel: string[] ["Netway Cal Template.xls", "ZGW Cal Template.xls"] -> [w402] mode=indexing
          tunnel: w382 -> [w401]
          tunnel: w381 -> [w400]
          tunnel: w380 -> [w396]
          tunnel: [w395] -> w367 mode=indexing
          n231 = Build Path(base path=w400, name or relative path=w402) -> (appended path=w395:path)
          n232 = Build Path(base path=w401, name or relative path=w402) -> (appended path=w397:path)
          n233 = call <vilib>:"Check if File or Folder Exists.vi"("error in (no error)"=w396, "path"=w395) -> ("file or folder exists?"=w399:bool, "dup path"=w398:path)  [unwired: 7 in, 1 out]
          n234 = case shown="False" w399 {
            tunnel: w398 -> [w404 _]
            tunnel: w397 -> [w403 _]
            frame False {
              n235 = Copy(10:w404, 11:w403) -> ()  [unwired: 3 in, 3 out]
            }
            frame True {
            }
          }
        }
        n236 = Index Array(array=w367) -> (element #1=w366:path, element #2=w365:path)  [unwired: 2 in]
        n237 = Bundle By Name(cluster=w385, "Cal Files Base Path"=w381, "Base Path"=w375, "Cal Targets Path"=w383, "Cal Template Path"=w366, "ZGW Template Path"=w365, "Firmware Version"="8.12.b5", "Software Version"="8.12.5" ("Firmware Version")) -> (w394:T7)
        n238 = local write "Cancel Output"(w370) -> ()
        n239 = local write "OK Output"(w370) -> ()
        n240 = local write "Netway"(0 ("Netway")) -> ()
        n241 = property on="Cal Table" class="Tbl (strict)"("Value"=string[][] [] ("Cal Table")) -> ()  [unwired: 2 in, 2 out]
      }
      frame "Unused Items" {
      }
      frame "Init Cal" {
        w408 = FALSE ("Verify Read")
        w411 = FALSE ("Auto")
        w407 = T9."Enabled" ("Disabled")
        w416 = T9."Disabled and Grayed Out" ("Disabled")
        w417 = T9."Disabled and Grayed Out" ("Disabled")
        n242 = Unbundle By Name(w420) -> ("Cal Log Header"=w418:string[])
        n243 = local write "Auto"(w408) -> ()
        n244 = local write "Verify Edit"(w408) -> ()
        n245 = property on="Cal Table" class="Tbl (strict)"("DisabledEnum"=w407) -> ()  [unwired: 2 in, 2 out]
        n246 = property on="Verify Read" class="Bool (strict)"("DisabledEnum"=w407) -> ()  [unwired: 2 in, 2 out]
        n247 = local write "Verify Read"(w408) -> ()
        n248 = property on="Cal Table" class="Tbl (strict)"("Column Headers[]"=w418) -> ()  [unwired: 2 in, 2 out]
        n249 = property on="Save Cal" class="Bool"("DisabledEnum"=w417) -> ()  [unwired: 2 in, 2 out]
        n250 = property on="Cancel Cal" class="Bool (strict)"("DisabledEnum"=w417) -> ()  [unwired: 2 in, 2 out]
        n251 = property on="Verify Tab" class="TabCtl (strict)"("Visible"=FALSE) -> ()  [unwired: 2 in, 2 out]
        n252 = property on="Hide Cal Values" class="Bool"("Visible"=TRUE) -> ()  [unwired: 2 in, 2 out]
        n253 = Insert Into Array(array=w413, index=0, new element=string[] ["Clear Dev Data", "Update Dev Tables", "Load Template"]) -> (w412:string[])
        n254 = property on="Reading Value 1" class="DigNum (strict)"("DisabledEnum"=w416) -> ()  [unwired: 2 in, 2 out]
        n255 = property on="Cal Value 1" class="DigNum (strict)"("DisabledEnum"=w416) -> ()  [unwired: 2 in, 2 out]
        n256 = property on="Confirm 1st Point" class="Bool (strict)"("DisabledEnum"=w416) -> ()  [unwired: 2 in, 2 out]
        n257 = property on="Reading Value 2" class="DigNum (strict)"("DisabledEnum"=w416) -> ()  [unwired: 2 in, 2 out]
        n258 = property on="Cal Value 2" class="DigNum (strict)"("DisabledEnum"=w416) -> ()  [unwired: 2 in, 2 out]
        n259 = property on="Confirm 2nd Point" class="Bool (strict)"("DisabledEnum"=w416) -> ()  [unwired: 2 in, 2 out]
        n260 = property on="Reading Value 3" class="DigNum (strict)"("DisabledEnum"=w416) -> ()  [unwired: 2 in, 2 out]
        n261 = property on="Cal Value 3" class="DigNum (strict)"("DisabledEnum"=w416) -> ()  [unwired: 2 in, 2 out]
        n262 = property on="Confirm 3rd Point" class="Bool (strict)"("DisabledEnum"=w416) -> ()  [unwired: 2 in, 2 out]
        n263 = property on="f(x)" class="DigNum (strict)"("DisabledEnum"=w416) -> ()  [unwired: 2 in, 2 out]
        n264 = property on="a0" class="DigNum (strict)"("DisabledEnum"=w416) -> ()  [unwired: 2 in, 2 out]
        n265 = property on="a1" class="DigNum (strict)"("DisabledEnum"=w416) -> ()  [unwired: 2 in, 2 out]
        n266 = property on="a2" class="DigNum (strict)"("DisabledEnum"=w416) -> ()  [unwired: 2 in, 2 out]
        n267 = Bundle By Name(cluster=w420, "Auto"=w411, "Review"=w411) -> (w419:T7)
      }
      frame "Adjust Channels" {
        n268 = Unbundle By Name(w428) -> ("ZGW?"=w421:bool, "Channel to Cal"=w425:T2, "Cal Unit"=w422:T3, "In/Out"=w424:T1)
        n269 = case shown="False" w421 {
          tunnel: [w440 w517] -> w426
          tunnel: w425 -> [w434 w511]
          tunnel: w424 -> [w433 w510]
          tunnel: [w432 w509] -> w423
          tunnel: w422 -> [w431 w508]
          frame True {
            # "ZGW."
            n270 = property on="Cal Unit" class="Enum (strict)"() -> ("Strings []"=w441:string[])  [unwired: 2 in, 2 out]
            n271 = property on="In/Out" class="Enum (strict)"() -> ("Strings []"=w439:string[])  [unwired: 2 in, 2 out]
            n272 = for {
              tunnel: w441 -> [w490] mode=indexing
              shift-right: [w488] -> w442
              shift-left: i32[] [] ("Disabled Items []") -> [w489]
              tunnel: w434 -> [w486]
              i -> [w487]
              n273 = case shown="\"%\", \"Hz\"" w490 {
                tunnel: w489 -> [w494 w502]
                tunnel: [w492 w500] -> w488
                tunnel: w487 -> [w493 w501]
                tunnel: w486 -> [w491 w499]
                frame "V", Default {
                  n274 = case shown="\"IO5\", \"IO6\", \"IO11\"..\"AIO8\"" w491 {
                    tunnel: w494 -> [w497 w498]
                    tunnel: w493 -> [w496 _]
                    tunnel: [w495 w498] -> w492
                    frame Default {
                      n275 = Build Array (concatenate)(w497, w496) -> (w495:i32[])
                    }
                    frame "IO5", "IO6", "IO11".."AIO8" {
                    }
                  }
                }
                frame "%", "Hz" {
                  n276 = case shown="\"IO5\", \"IO6\"" w499 {
                    tunnel: w502 -> [w505 w506]
                    tunnel: w501 -> [w504 _]
                    tunnel: [w503 w506] -> w500
                    frame Default {
                      n277 = Build Array (concatenate)(w505, w504) -> (w503:i32[])
                    }
                    frame "IO5", "IO6" {
                    }
                  }
                }
              }
            }
            n278 = for {
              tunnel: w439 -> [w459] mode=indexing
              shift-right: [w457] -> w438
              shift-left: i32[] [] ("Disabled Items []") -> [w458]
              tunnel: w434 -> [w455]
              tunnel: w431 -> [w454]
              i -> [w456]
              n279 = case shown="\"Output\"" w459 {
                tunnel: w458 -> [w460 w465]
                tunnel: [w460 w463] -> w457
                tunnel: w456 -> [_ w464]
                tunnel: w455 -> [_ w462]
                tunnel: w454 -> [_ w461]
                frame "Input", Default {
                }
                frame "Output" {
                  n280 = case shown="\"IO1\"..\"IO8\", Default" w462 {
                    tunnel: w465 -> [w468 w476 w477]
                    tunnel: w464 -> [w467 w475 _]
                    tunnel: [w466 w474 w477] -> w463
                    tunnel: w461 -> [w469 _ _]
                    frame "IO1".."IO8", Default {
                      n281 = case shown="\"V\", Default" w469 {
                        tunnel: w468 -> [w472 w473]
                        tunnel: w467 -> [w471 _]
                        tunnel: [w470 w473] -> w466
                        frame "V", Default {
                          n282 = Build Array (concatenate)(w472, w471) -> (w470:i32[])
                        }
                        frame "%", "Hz" {
                        }
                      }
                    }
                    frame "IO9".."IO12" {
                      n283 = Build Array (concatenate)(w476, w475) -> (w474:i32[])
                    }
                    frame "AIO1".."AIO8" {
                    }
                  }
                }
              }
            }
            n284 = property on="Channel to Cal" class="Enum (strict)"("Disabled Items []"=i32[] [0, 1, 2, 3, 6, 7, 8, 9]) -> ()  [unwired: 2 in, 2 out]
            n285 = property on="Cal Unit" class="Enum (strict)"("Disabled Items []"=w442) -> ()  [unwired: 2 in, 2 out]
            n286 = property on="In/Out" class="Enum (strict)"("Disabled Items []"=w438) -> ()  [unwired: 2 in, 2 out]
            n287 = Search 1D Array(1D array=w442, element=w431) -> (index of element=w443:i32)  [unwired: 1 in]
            n288 = Search 1D Array(1D array=w438, element=w433) -> (index of element=w437:i32)  [unwired: 1 in]
            n289 = Greater Or Equal To 0?(x=w443) -> (x >= 0?=w444:bool)
            n290 = Greater Or Equal To 0?(x=w437) -> (x >= 0?=w436:bool)
            n291 = case shown="True" w444 {
              tunnel: [w478 w479] -> w440
              tunnel: w431 -> [w478 _]
              tunnel: w442 -> [_ w481]
              frame False {
              }
              frame True {
                n292 = for {
                  N: 3 -> [_]
                  tunnel: w481 -> [w485]
                  tunnel: [w482] -> w479
                  i -> [w482]
                  stop <- w483 stop-if-true
                  n293 = Search 1D Array(1D array=w485, element=w482) -> (index of element=w484:i32)  [unwired: 1 in]
                  n294 = Less Than 0?(x=w484) -> (x < 0?=w483:bool)
                }
                n295 = local write "Cal Unit"(w479) -> ()
              }
            }
            n296 = case shown="True" w436 {
              tunnel: [w446 w447] -> w432
              tunnel: w433 -> [w446 _]
              tunnel: w438 -> [_ w449]
              frame False {
              }
              frame True {
                n297 = for {
                  N: 2 -> [_]
                  tunnel: w449 -> [w453]
                  tunnel: [w450] -> w447
                  i -> [w450]
                  stop <- w451 stop-if-true
                  n298 = Search 1D Array(1D array=w453, element=w450) -> (index of element=w452:i32)  [unwired: 1 in]
                  n299 = Less Than 0?(x=w452) -> (x < 0?=w451:bool)
                }
                n300 = local write "In/Out"(w447) -> ()
              }
            }
          }
          frame False {
            # "Netway."
            n301 = property on="Cal Unit" class="Enum (strict)"() -> ("Strings []"=w518:string[])  [unwired: 2 in, 2 out]
            n302 = property on="In/Out" class="Enum (strict)"() -> ("Strings []"=w516:string[])  [unwired: 2 in, 2 out]
            n303 = for {
              tunnel: w518 -> [w567] mode=indexing
              shift-right: [w565] -> w519
              shift-left: i32[] [] ("Disabled Items []") -> [w566]
              tunnel: w511 -> [w563]
              i -> [w564]
              n304 = case shown="\"%\", \"Hz\"" w567 {
                tunnel: w566 -> [w568 w572]
                tunnel: [w568 w570] -> w565
                tunnel: w564 -> [_ w571]
                tunnel: w563 -> [_ w569]
                frame "V", Default {
                }
                frame "%", "Hz" {
                  n305 = case shown="\"IO1\"..\"IO8\", Default" w569 {
                    tunnel: w572 -> [w575 w576]
                    tunnel: w571 -> [w574 _]
                    tunnel: [w573 w576] -> w570
                    frame "IO9".."AIO8" {
                      n306 = Build Array (concatenate)(w575, w574) -> (w573:i32[])
                    }
                    frame "IO1".."IO8", Default {
                    }
                  }
                }
              }
            }
            n307 = for {
              tunnel: w516 -> [w536] mode=indexing
              shift-right: [w534] -> w515
              shift-left: i32[] [] ("Disabled Items []") -> [w535]
              tunnel: w511 -> [w532]
              tunnel: w508 -> [w531]
              i -> [w533]
              n308 = case shown="\"Output\"" w536 {
                tunnel: w535 -> [w537 w542]
                tunnel: [w537 w540] -> w534
                tunnel: w533 -> [_ w541]
                tunnel: w532 -> [_ w539]
                tunnel: w531 -> [_ w538]
                frame "Input", Default {
                }
                frame "Output" {
                  n309 = case shown="\"IO1\"..\"IO8\", Default" w539 {
                    tunnel: w542 -> [w545 w553 w554]
                    tunnel: w541 -> [w544 w552 _]
                    tunnel: [w543 w551 w554] -> w540
                    tunnel: w538 -> [w546 _ _]
                    frame "IO1".."IO8", Default {
                      n310 = case shown="\"V\", Default" w546 {
                        tunnel: w545 -> [w549 w550]
                        tunnel: w544 -> [w548 _]
                        tunnel: [w547 w550] -> w543
                        frame "V", Default {
                          n311 = Build Array (concatenate)(w549, w548) -> (w547:i32[])
                        }
                        frame "%", "Hz" {
                        }
                      }
                    }
                    frame "IO9".."IO12" {
                      n312 = Build Array (concatenate)(w553, w552) -> (w551:i32[])
                    }
                    frame "AIO1".."AIO8" {
                    }
                  }
                }
              }
            }
            n313 = property on="Channel to Cal" class="Enum (strict)"("Disabled Items []"=i32[] []) -> ()  [unwired: 2 in, 2 out]
            n314 = property on="Cal Unit" class="Enum (strict)"("Disabled Items []"=w519) -> ()  [unwired: 2 in, 2 out]
            n315 = property on="In/Out" class="Enum (strict)"("Disabled Items []"=w515) -> ()  [unwired: 2 in, 2 out]
            n316 = Search 1D Array(1D array=w519, element=w508) -> (index of element=w520:i32)  [unwired: 1 in]
            n317 = Search 1D Array(1D array=w515, element=w510) -> (index of element=w514:i32)  [unwired: 1 in]
            n318 = Greater Or Equal To 0?(x=w520) -> (x >= 0?=w521:bool)
            n319 = Greater Or Equal To 0?(x=w514) -> (x >= 0?=w513:bool)
            n320 = case shown="True" w521 {
              tunnel: [w555 w556] -> w517
              tunnel: w508 -> [w555 _]
              tunnel: w519 -> [_ w558]
              frame False {
              }
              frame True {
                n321 = for {
                  N: 3 -> [_]
                  tunnel: w558 -> [w562]
                  tunnel: [w559] -> w556
                  i -> [w559]
                  stop <- w560 stop-if-true
                  n322 = Search 1D Array(1D array=w562, element=w559) -> (index of element=w561:i32)  [unwired: 1 in]
                  n323 = Less Than 0?(x=w561) -> (x < 0?=w560:bool)
                }
                n324 = local write "Cal Unit"(w556) -> ()
              }
            }
            n325 = case shown="True" w513 {
              tunnel: [w523 w524] -> w509
              tunnel: w510 -> [w523 _]
              tunnel: w515 -> [_ w526]
              frame False {
              }
              frame True {
                n326 = for {
                  N: 2 -> [_]
                  tunnel: w526 -> [w530]
                  tunnel: [w527] -> w524
                  i -> [w527]
                  stop <- w528 stop-if-true
                  n327 = Search 1D Array(1D array=w530, element=w527) -> (index of element=w529:i32)  [unwired: 1 in]
                  n328 = Less Than 0?(x=w529) -> (x < 0?=w528:bool)
                }
                n329 = local write "In/Out"(w524) -> ()
              }
            }
          }
        }
        n330 = Bundle By Name(cluster=w428, "Cal Unit"=w426, "In/Out"=w423) -> (w427:T7)
      }
      frame "Button State" {
        n331 = Unbundle By Name(w579) -> ("Init"=w577:bool, "Cal Unit"=w580:T3)
        n332 = case shown="False" w577 {
          tunnel: w580 -> [w581 _]
          frame False {
            n333 = case shown="Default" w581 {
              tunnel: [T9."Enabled" ("Disabled") T9."Disabled and Grayed Out" ("Disabled")] -> w582
              frame Default {
              }
              frame "%", "Hz" {
              }
            }
            n334 = property on="Start Cal" class="Bool"("DisabledEnum"=w582) -> ()  [unwired: 2 in, 2 out]
          }
          frame True {
          }
        }
      }
      frame "Clear Dev Data" {
        n335 = Bundle By Name(cluster=w586, "Verify Table"=string[][] [["", "", "", "", ""], ["", "", "", "", ""], ["", "", "", "", ""], ["", "", "", "", ""], ["", "", "", "", ""], ["", "", "", "", ""], ["", "", "", "", ""], ["", "", "", "", ""], ["", "", "", "", ""], ["", "", "", "", ""]]) -> (w585:T7)
      }
      frame "Update Dev Tables" {
        n336 = Unbundle By Name(w590) -> ("Verify Table"=w589:string[][])
        n337 = local write "Verify Table"(w589) -> ()
      }
      frame "Load Template" {
        n338 = Unbundle By Name(w594) -> ("Cal Template Path"=w598:path)
        n339 = call <vilib>:"Check if File or Folder Exists.vi"("path"=w598) -> ("file or folder exists?"=w599:bool)  [unwired: 8 in, 2 out]
        n340 = case shown="True" w599 {
          tunnel: [string[] [] string[] []] -> w600
          tunnel: w598 -> [w605 w616]
          tunnel: [FALSE ("Visible") FALSE ("Visible")] -> w597
          tunnel: [w602 w608] -> w596
          tunnel: [w602 w608] -> w595
          frame False {
            w602 = T9."Disabled and Grayed Out" ("Disabled")
            n341 = Format Into String(format string="Can't find cal spreadsheet template!\n\nShould have been here:  \"%s\"" ("message"), w605) -> (resulting string=w604:string)  [unwired: 2 in, 1 out]
            n342 = One Button Dialog(message=w604) -> ()  [unwired: 1 in, 1 out]
          }
          frame True {
            w608 = T9."Enabled" ("Disabled")
            n343 = call "Read Write Header.vi"("Cal Template Path"=w616, "Write (F)"=FALSE) -> ("Header Table 1"=w615:string[][], "Header Table 2"=w614:string[][], "Sys Cal Table"=w611:string[][], "Cal Standards Table"=w610:string[][], "Header Comments"=w612:string[][])  [unwired: 13 in]
            n344 = local write "Header Comments"(w612) -> ()
            n345 = local write "Sys Cal Table"(w611) -> ()
            n346 = local write "Cal Standards Table"(w610) -> ()
            n347 = local write "Header Table 1"(w615) -> ()
            n348 = local write "Header Table 2"(w614) -> ()
          }
        }
        n349 = property on="Load Indicator Tab" class="TabCtl (strict)"("Visible"=w597) -> ()  [unwired: 2 in, 2 out]
        n350 = property on="Header OK" class="Bool"("DisabledEnum"=w596) -> ()  [unwired: 2 in, 2 out]
        n351 = property on="Header Cancel" class="Bool"("DisabledEnum"=w595) -> ()  [unwired: 2 in, 2 out]
        n352 = Insert Into Array(array=w593, index=0, new element=w600) -> (w592:string[])
      }
      frame "Create Spreadsheet" {
        n353 = Unbundle By Name(w625) -> ("ZGW Template Path"=w620:path, "ZGW?"=w621:bool, "Cal Template Path"=w619:path, "Netway"=w635:i32, "Cal Files Base Path"=w631:path)
        n354 = Select(t=w620, s=w621, f=w619) -> (s? t:f=w618:path)
        n355 = Format Into String(format string="%04d.xls" ("initial string"), w635) -> (resulting string=w630:string)  [unwired: 2 in, 1 out]
        n356 = Build Path(base path=w631, name or relative path=w630) -> (appended path=w629:path)
        n357 = Not A Number/Path/Refnum?(number/path/refnum=w629) -> (NaN/Path/Refnum?=w628:bool)
        n358 = Equal To 0?(x=w635) -> (x = 0?=w627:bool)
        n359 = Or(x=w628, y=w627) -> (x .or. y?=w626:bool)
        n360 = case shown="False" w626 {
          tunnel: [string[] ["Save Header"] string[] []] -> w632
          tunnel: w629 -> [w637 _]
          tunnel: w618 -> [w638 _]
          frame False {
            n361 = call <vilib>:"Check if File or Folder Exists.vi"("path"=w637) -> ("file or folder exists?"=w640:bool)  [unwired: 8 in, 2 out]
            n362 = case shown="True" w640 {
              tunnel: [FALSE ("T button?") w644] -> w639
              frame False {
              }
              frame True {
                n363 = Two Button Dialog(message="Cal file already exists.  How do you want to proceed?\n\n\"Use Existing\" will continue with existing file and data.  \"Overwrite\" will destroy all data and start with fresh template", 1:"Overwrite" ("F button name (\"Cancel\")"), 2:"Use Existing" ("T button name (\"OK\")")) -> (T button?=w644:bool)
              }
            }
            n364 = case shown="False" w639 {
              tunnel: w637 -> [w648 _]
              tunnel: w638 -> [w647 _]
              frame False {
                n365 = Copy(9:TRUE ("overwrite (F)"), 10:w648, 11:w647) -> ()  [unwired: 2 in, 3 out]
              }
              frame True {
              }
            }
          }
          frame True {
            w649 = T9."Enabled" ("Disabled")
            n366 = property on="Load Indicator Tab" class="TabCtl (strict)"("Visible"=FALSE) -> ()  [unwired: 2 in, 2 out]
            n367 = property on="Header OK" class="Bool"("DisabledEnum"=w649) -> ()  [unwired: 2 in, 2 out]
            n368 = property on="Header Cancel" class="Bool"("DisabledEnum"=w649) -> ()  [unwired: 2 in, 2 out]
            n369 = One Button Dialog(message="\"Manufacturer Serial #\" is blank or contains invalid characters.") -> ()  [unwired: 1 in, 1 out]
          }
        }
        n370 = Bundle By Name(cluster=w625, "Cal Spreadsheet Path"=w629) -> (w622:T7)
        n371 = Insert Into Array(array=w624, index=0, new element=w632) -> (w623:string[])
      }
      frame "Save Header" {
        n372 = Unbundle By Name(w660) -> ("Cal Spreadsheet Path"=w663:path, "Cal Template Path"=w662:path)
        n373 = Build Array(w663, w662) -> (w661:path[])
        n374 = for {
          tunnel: "Header Table 2" -> [w674]
          tunnel: "Sys Cal Table" -> [w673]
          tunnel: "Cal Standards Table" -> [w672]
          tunnel: "Header Comments" -> [w671]
          tunnel: [w670] -> w664
          tunnel: "Header Table 1" -> [w668]
          tunnel: w661 -> [w667] mode=indexing
          n375 = call "Read Write Header.vi"("Header Table 1 IN"=w668, "Header Table 2 IN"=w674, "Sys Cal Table IN"=w673, "Cal Standards Table IN"=w672, "Header Comments IN"=w671, "Cal Template Path"=w667, "Write (F)"=TRUE) -> ("Header Table 1"=w670:string[][])  [unwired: 8 in, 4 out]
        }
        n376 = flat-sequence {
          tunnel: w664 -> [_]
          frame #0 {
            w675 = T9."Enabled" ("Disabled")
            w676 = FALSE ("Visible")
            n377 = property on="View Spreadsheet" class="Bool"("DisabledEnum"=w675) -> ()  [unwired: 2 in, 2 out]
            n378 = property on="Main Tab" class="TabCtl (strict)"("DisabledEnum"=w675) -> ()  [unwired: 2 in, 2 out]
            n379 = property on="Netway" class="DigNum (strict)"("DisabledEnum"=w675) -> ()  [unwired: 2 in, 2 out]
            n380 = property on="Channel to Cal" class="Enum (strict)"("DisabledEnum"=w675) -> ()  [unwired: 2 in, 2 out]
            n381 = property on="Cal Unit" class="Enum (strict)"("DisabledEnum"=w675) -> ()  [unwired: 2 in, 2 out]
            n382 = property on="Start Cal" class="Bool"("DisabledEnum"=w675) -> ()  [unwired: 2 in, 2 out]
            n383 = property on="Start Verification" class="Bool"("DisabledEnum"=w675) -> ()  [unwired: 2 in, 2 out]
            n384 = property on="In/Out" class="Enum (strict)"("DisabledEnum"=w675) -> ()  [unwired: 2 in, 2 out]
            n385 = property on="Load Indicator Tab" class="TabCtl (strict)"("Visible"=w676) -> ()  [unwired: 2 in, 2 out]
            n386 = property on="Header Tab" class="TabCtl (strict)"("Visible"=w676) -> ()  [unwired: 2 in, 2 out]
          }
        }
        n387 = Insert Into Array(array=w659, index=0, new element=string[] []) -> (w658:string[])
      }
      frame "Load Coefficients" {
        n388 = Unbundle By Name(w682) -> ("Netway"=w681:i32)
        n389 = call "Read ALL Cal Parameters.vi"("Serial Number"=w681) -> ("Error OUT"=w680:errorcluster, "a2"=w677:dbl[], "a1"=w678:dbl[], "a0"=w679:dbl[])  [unwired: 7 in]
        n390 = case shown="No Error" w680 {
          tunnel: [string[] [] string[] ["End Cal"]] -> w685
          tunnel: w679 -> [w696 _]
          tunnel: w678 -> [w695 _]
          tunnel: w677 -> [w694 _]
          frame No Error {
            w697 = i16 8 ("precision (6)")
            n391 = Number To Fractional String(number=w696, precision (6)=w697) -> (F-format string=w691:string[])  [unwired: 2 in]
            n392 = Number To Fractional String(number=w695, precision (6)=w697) -> (F-format string=w690:string[])  [unwired: 2 in]
            n393 = Number To Fractional String(number=w694, precision (6)=w697) -> (F-format string=w689:string[])  [unwired: 2 in]
            n394 = Transpose 2D Array(2D array=string[][] [["IO1", "V", "Input"], ["IO2", "V", "Input"], ["IO3", "V", "Input"], ["IO4", "V", "Input"], ["IO5", "V", "Input"], ["IO6", "V", "Input"], ["IO7", "V", "Input"], ["IO8", "V", "Input"], ["IO9", "V", "Input"], ["IO10", "V", "Input"], ["IO11", "V", "Input"], ["IO12", "V", "Input"], ["AIO1", "V", "Input"], ["AIO2", "V", "Input"], ["AIO3", "V", "Input"], ["AIO4", "V", "Input"], ["AIO5", "V", "Input"], ["AIO6", "V", "Input"], ["AIO7", "V", "Input"], ["AIO8", "V", "Input"], ["AIO1", "V", "Output"], ["AIO2", "V", "Output"], ["AIO3", "V", "Output"], ["AIO4", "V", "Output"], ["AIO5", "V", "Output"], ["AIO6", "V", "Output"], ["AIO7", "V", "Output"], ["AIO8", "V", "Output"]]) -> (transposed array=w692:string[][])
            n395 = Build Array (concatenate)(w692, w691, w690, w689) -> (w688:string[][])
            n396 = Transpose 2D Array(2D array=w688) -> (transposed array=→"Cal Table":string[][])
          }
          frame Error {
            n397 = One Button Dialog(message="Failed to load calibration coefficients.  Calibration will now be terminated.") -> ()  [unwired: 1 in, 1 out]
          }
        }
        n398 = Insert Into Array(array=w684, index=0, new element=w685) -> (w683:string[])
      }
      frame "Load Targets" {
        w705 = T9."Disabled and Grayed Out" ("Disabled")
        n399 = Unbundle By Name(w716) -> ("Cal Targets Path"=w720:path, "Targets"=w725:T4, "Cal Unit"=w727:T3, "Channel to Cal"=w707:T2, "In/Out"=w706:T1, "Verify Table"=w717:string[][])
        n400 = property on="Cancel Cal" class="Bool (strict)"("DisabledEnum"=T9."Enabled" ("Disabled")) -> ()  [unwired: 2 in, 2 out]
        n401 = property on="Cal Table" class="Tbl (strict)"("Active Cell"=T10 {"Row"=-2, "Column"=-2} ("Active Cell:Active Cell"), "Cell BG Color"=u32 16448250) -> ()  [unwired: 2 in, 2 out]
        n402 = call <vilib>:"Open Config Data.vi"("configuration file path"=w720) -> ("error out"=w722:errorcluster, "refnum"=w721:T12)  [unwired: 8 in, 1 out]
        n403 = call <userlib>:"Read INI Cluster__ogtk.vi"("error in (no error)"=w722, "INI Fomatted Cluster Type"=w725, "refnum"=w721) -> ("error out"=w724:errorcluster, "INI Fomatted Cluster"=w726:variant, "dup refnum"=w723:T12)  [unwired: 4 in, 2 out]
        n404 = property on="Netway" class="DigNum (strict)"("DisabledEnum"=w705) -> ()  [unwired: 2 in, 2 out]
        n405 = property on="Channel to Cal" class="Enum (strict)"("DisabledEnum"=w705) -> ()  [unwired: 2 in, 2 out]
        n406 = property on="Cal Unit" class="Enum (strict)"("DisabledEnum"=w705) -> ()  [unwired: 2 in, 2 out]
        n407 = property on="In/Out" class="Enum (strict)"("DisabledEnum"=w705) -> ()  [unwired: 2 in, 2 out]
        n408 = property on="Start Cal" class="Bool"("DisabledEnum"=w705) -> ()  [unwired: 2 in, 2 out]
        n409 = property on="Start Verification" class="Bool"("DisabledEnum"=w705) -> ()  [unwired: 2 in, 2 out]
        n410 = call <vilib>:"Close Config Data.vi"("error in (no error)"=w724, "refnum"=w723) -> ()  [unwired: 8 in, 2 out]
        n411 = Variant To Data(type=w725, Variant=w726) -> (data=w728:T4)  [unwired: 1 in, 1 out]
        n412 = case shown="\"Hz\"" w727 {
          tunnel: w728 -> [w743 w760 w770]
          tunnel: [w742 w759 w769] -> w729
          tunnel: [w741 w758 w768] -> w731
          tunnel: w707 -> [w740 _ _]
          tunnel: w706 -> [w739 w757 w767]
          frame "V", Default {
            n413 = case shown="\"AIO1\"..\"AIO8\"" w740 {
              tunnel: w743 -> [w746 w750]
              tunnel: [w745 w749] -> w742
              tunnel: [w744 w748] -> w741
              tunnel: w739 -> [_ w747]
              frame "IO1".."IO12", Default {
                n414 = Unbundle By Name(w746) -> ("V0-11"=w745:T5, "AI0-11 Setpoints"=w744:T6)
              }
              frame "AIO1".."AIO8" {
                n415 = case shown="\"Output\"" w747 {
                  tunnel: w750 -> [w753 w756]
                  tunnel: [w752 w755] -> w749
                  tunnel: [w751 w754] -> w748
                  frame "Input", Default {
                    n416 = Unbundle By Name(w753) -> ("V12-19"=w752:T5, "AI12-19 Setpoints"=w751:T6)
                  }
                  frame "Output" {
                    n417 = Unbundle By Name(w756) -> ("AO"=w755:T5, "AI12-19 Setpoints"=w754:T6)
                  }
                }
              }
            }
          }
          frame "%" {
            n418 = case shown="\"Output\"" w757 {
              tunnel: w760 -> [w763 w766]
              tunnel: [w762 w765] -> w759
              tunnel: [w761 w764] -> w758
              frame "Input", Default {
                n419 = Unbundle By Name(w763) -> ("%"=w762:T5, "Duty Setpoints"=w761:T6)
              }
              frame "Output" {
                n420 = Unbundle By Name(w766) -> ("%_out"=w765:T5, "Duty Setpoints"=w764:T6)
              }
            }
          }
          frame "Hz" {
            n421 = case shown="\"Output\"" w767 {
              tunnel: w770 -> [w773 w776]
              tunnel: [w772 w775] -> w769
              tunnel: [w771 w774] -> w768
              frame "Input", Default {
                n422 = Unbundle By Name(w773) -> ("Hz"=w772:T5, "Hz Setpoints"=w771:T6)
              }
              frame "Output" {
                n423 = Unbundle By Name(w776) -> ("Hz_out"=w775:T5, "Hz Setpoints"=w774:T6)
              }
            }
          }
        }
        n424 = Cluster To Array(cluster=w729) -> (array=w733:dbl[])
        n425 = Cluster To Array(cluster=w731) -> (array=w732:dbl[])
        n426 = Delete From Array(array=w733, length=1, index=0 ("length")) -> (deleted portion=w737:dbl[], array with subset deleted=w735:dbl[])
        n427 = call-poly <userlib>:"Remove Duplicates from 1D Array__ogtk.vi"("Input Array"=w735) -> ("Output Array"=w703:dbl[])  [unwired: 1 out]
        n428 = call-poly <userlib>:"Filter 1D Array__ogtk.vi"("items to filter"=dbl[] [0.0], "array"=w703) -> ("filtered array"=w701:dbl[])  [unwired: 4 in, 1 out]
        n429 = Build Array (concatenate)(w737, w701) -> (w736:dbl[])
        n430 = Number To Fractional String(number=w736, precision (6)=i16 3) -> (F-format string=w730:string[])  [unwired: 2 in]
        n431 = Index Array(array=w732) -> (element #1=w714:dbl, element #2=w713:dbl, element #3=w712:dbl)  [unwired: 3 in]
        n432 = Replace Array Subset(array=w717, new element=w730, index (col)=0 ("disabled index (col)")) -> (w719:string[][])  [unwired: 1 in]
        n433 = local write "Cal Value 1"(w714) -> ()
        n434 = local write "Cal Value 2"(w713) -> ()
        n435 = local write "Cal Value 3"(w712) -> ()
        n436 = Bundle By Name(cluster=w716, "Targets"=w728, "Verify Table"=w719) -> (w715:T7)
        n437 = property on="Verify Table" class="Tbl (strict)"("Value"=w719) -> ()  [unwired: 2 in, 2 out]
      }
      frame "Init Coeffs" {
        n438 = Unbundle By Name(w783) -> ("Netway"=w782:i32, "Channel to Cal"=w781:T2, "In/Out"=w780:T1)
        n439 = call "Write Cal Parameters.vi"("Serial Number"=w782, "Store (T)"=FALSE, "a0"=0.0, "a1"=1.0 ("a0"), "a2"=0.0 ("a0"), "Channel"=w781, "In/Out"=w780) -> ("Error OUT"=w779:errorcluster)  [unwired: 8 in]
        n440 = case shown="Error" w779 {
          tunnel: [w788 string[] []] -> w777
          tunnel: w778 -> [w788 _]
          frame No Error {
          }
          frame Error {
            n441 = One Button Dialog(message="Failed to initialize coefficients on Netway.  Calibration for this channel will now be terminated.") -> ()  [unwired: 1 in, 1 out]
          }
        }
      }
      frame "Start Cal" {
        w797 = T9."Enabled" ("Disabled")
        n442 = Unbundle By Name(w795) -> ("DMM Connected"=w792:bool, "Cal Unit"=w793:T3, "In/Out"=w791:T1)
        n443 = property on="Reading Value 1" class="DigNum (strict)"("DisabledEnum"=w797) -> ()  [unwired: 2 in, 2 out]
        n444 = property on="Cal Value 1" class="DigNum (strict)"("DisabledEnum"=w797) -> (error out=w798:errorcluster)  [unwired: 2 in, 1 out]
        n445 = property on="Confirm 1st Point" class="Bool (strict)"("DisabledEnum"=w797) -> ()  [unwired: 2 in, 2 out]
        n446 = property on="Cancel Cal" class="Bool (strict)"("DisabledEnum"=w797) -> ()  [unwired: 2 in, 2 out]
        n447 = property on="Cal Value 1" class="DigNum (strict)"(error in=w798, "Key Focus"=TRUE) -> ()  [unwired: 1 in, 2 out]
        n448 = case shown="\"Output\"" w791 {
          tunnel: [string[] ["First Cal Point"] string[] ["Set Output", "First Cal Point"]] -> w802
          tunnel: w795 -> [w803 w810]
          tunnel: [w803 w806] -> w794
          tunnel: w793 -> [_ w808]
          tunnel: w792 -> [_ w805]
          frame "Input", Default {
          }
          frame "Output" {
            n449 = Bundle By Name(cluster=w810, "Output Index"=u8 0) -> (w807:T7)
            n450 = case shown="\"V\"" w808 {
              tunnel: w807 -> [w815 w821]
              tunnel: [w814 w821] -> w806
              tunnel: w805 -> [w813 _]
              frame "V" {
                n451 = case shown="False" w813 {
                  selector: w813 -> [_ w820]
                  tunnel: [w816 w820] -> w812
                  frame False {
                    n452 = call "Keithly 2000 Global.vi"("Mode (Read)"=enum16{"Init", "Read DC Volts", "Close"}."Init", "GPIB Reference"=refnum<visa-resource-name> "GPIB0::16::INSTR") -> ("error out"=w817:errorcluster)  [unwired: 8 in, 1 out]
                    n453 = Not(x=w817) -> (.not. x?=w816:bool)
                  }
                  frame True {
                  }
                }
                n454 = Bundle By Name(cluster=w815, "DMM Connected"=w812) -> (w814:T7)
              }
              frame Default {
              }
            }
          }
        }
        n455 = Insert Into Array(array=w800, index=0, new element=w802) -> (w801:string[])
      }
      frame "Set Output" {
        n456 = Unbundle By Name(w829) -> ("Review"=w823:bool, "Targets"=w825:T4, "Output Index"=w824:u8, "Netway"=w828:i32, "Channel to Cal"=w827:T2, "Cal Unit"=w826:T3, "In/Out"=w822:T1)
        n457 = case shown="\"Output\"" w822 {
          tunnel: w828 -> [_ w836]
          tunnel: w827 -> [_ w835]
          tunnel: w826 -> [_ w834]
          tunnel: w825 -> [_ w833]
          tunnel: w824 -> [_ w832]
          tunnel: w823 -> [_ w831]
          frame "Input", Default {
          }
          frame "Output" {
            n458 = case shown="\"V\", Default" w834 {
              tunnel: w836 -> [w852 w865 w880]
              tunnel: w835 -> [w848 w862 w878]
              tunnel: w833 -> [w845 w860 w877]
              tunnel: w832 -> [w843 w859 w876]
              tunnel: w831 -> [w838 w854 w869]
              frame "V", Default {
                n459 = Unbundle By Name(w845) -> ("AO"=w841:T5, "AI12-19 Setpoints"=w844:T6)
                n460 = Cluster To Array(cluster=w841) -> (array=w840:dbl[])
                n461 = Cluster To Array(cluster=w844) -> (array=w839:dbl[])
                n462 = Select(t=w840, s=w838, f=w839) -> (s? t:f=w837:dbl[])
                n463 = Index Array(array=w837, index=w843) -> (element=w842:dbl)
                n464 = Multiply(x=w842, y=1000.0) -> (x*y=w850:dbl)
                n465 = Subtract(x=w848, y=u16 11) -> (x-y=w846:u16)
                n466 = To Long Integer(number=w850) -> (32bit integer=w849:i32)
                n467 = call "Write Analog Outputs.vi"("Value"=w849, "Analog Output"=w846, "Serial Number"=w852) -> ()  [unwired: 8 in, 1 out]
              }
              frame "%" {
                n468 = Unbundle By Name(w860) -> ("%_out"=w857:T5, "Duty Setpoints"=w861:T6)
                n469 = Cluster To Array(cluster=w857) -> (array=w856:dbl[])
                n470 = Cluster To Array(cluster=w861) -> (array=w855:dbl[])
                n471 = Select(t=w856, s=w854, f=w855) -> (s? t:f=w853:dbl[])
                n472 = Index Array(array=w853, index=w859) -> (element=w858:dbl)
                n473 = To Long Integer(number=w858) -> (32bit integer=w864:i32)
                n474 = case shown="Default" w864 {
                  tunnel: [1000 ("Frequency") 0 ("Frequency")] -> w863
                  frame Default {
                  }
                  frame 0 {
                  }
                }
                n475 = call "Write Pwm Outputs.vi"("Serial Number"=w865, "Output"=w862, "Duty"=w864, "Frequency"=w863) -> ()  [unwired: 11 in, 1 out]
              }
              frame "Hz" {
                n476 = Unbundle By Name(w877) -> ("Hz_out"=w872:T5, "Hz Setpoints"=w873:T6)
                n477 = Cluster To Array(cluster=w872) -> (array=w871:dbl[])
                n478 = Cluster To Array(cluster=w873) -> (array=w870:dbl[])
                n479 = Select(t=w871, s=w869, f=w870) -> (s? t:f=w868:dbl[])
                n480 = Index Array(array=w868, index=w876) -> (element=w875:dbl)
                n481 = To Long Integer(number=w875) -> (32bit integer=w874:i32)
                n482 = call "Write Pwm Outputs.vi"("Serial Number"=w880, "Output"=w878, "Duty"=50 ("Frequency"), "Frequency"=w874) -> ()  [unwired: 11 in, 1 out]
              }
            }
          }
        }
      }
      frame "First Cal Point" {
        n483 = Unbundle By Name(w890) -> ("Netway"=w889:i32, "Channel to Cal"=w888:T2, "Cal Unit"=w887:T3, "In/Out"=w886:T1, "DMM Connected"=w885:bool)
        n484 = call "Get Cal Point.vi"("Netway"=w889, "Channel to Cal"=w888, "Cal Unit"=w887, "In/Out"=w886, "DMM Connected in"=w885, "avg"="avg") -> ("DMM Connected out"=w883:bool, "Output Reading"=w881:bool, "Reading"=→"Reading Value 1":dbl)  [unwired: 7 in]
        n485 = case shown="True" w881 {
          selector: w881 -> [_ w896]
          frame False {
          }
          frame True {
            n486 = property on="Confirm 1st Point" class="Bool (strict)"("Val(Sgnl)"=w896) -> ()  [unwired: 2 in, 2 out]
          }
        }
        n487 = Bundle By Name(cluster=w890, "DMM Connected"=w883, "Output Reading"=w881) -> (w891:T7)
        n488 = Insert Into Array(array=w893, index=0, new element=string[] ["Main", "First Cal Point"]) -> (w894:string[])
      }
      frame "Second Cal Point" {
        n489 = Unbundle By Name(w901) -> ("Netway"=w907:i32, "Channel to Cal"=w906:T2, "Cal Unit"=w905:T3, "In/Out"=w904:T1, "DMM Connected"=w903:bool)
        n490 = local read "avg"() -> (w899:i32)
        n491 = call "Get Cal Point.vi"("Netway"=w907, "Channel to Cal"=w906, "Cal Unit"=w905, "In/Out"=w904, "DMM Connected in"=w903, "avg"=w899) -> ("DMM Connected out"=w902:bool, "Output Reading"=w897:bool, "Reading"=→"Reading Value 2":dbl)  [unwired: 7 in]
        n492 = case shown="True" w897 {
          selector: w897 -> [_ w912]
          frame False {
          }
          frame True {
            n493 = property on="Confirm 2nd Point" class="Bool (strict)"("Val(Sgnl)"=w912) -> ()  [unwired: 2 in, 2 out]
          }
        }
        n494 = Bundle By Name(cluster=w901, "DMM Connected"=w902, "Output Reading"=w897) -> (w900:T7)
        n495 = Insert Into Array(array=w908, index=0, new element=string[] ["Main", "Second Cal Point"]) -> (w909:string[])
      }
      frame "Final Cal Point" {
        n496 = Unbundle By Name(w917) -> ("Netway"=w923:i32, "Channel to Cal"=w922:T2, "Cal Unit"=w921:T3, "In/Out"=w920:T1, "DMM Connected"=w919:bool)
        n497 = local read "avg"() -> (w915:i32)
        n498 = call "Get Cal Point.vi"("Netway"=w923, "Channel to Cal"=w922, "Cal Unit"=w921, "In/Out"=w920, "DMM Connected in"=w919, "avg"=w915) -> ("DMM Connected out"=w918:bool, "Output Reading"=w913:bool, "Reading"=→"Reading Value 3":dbl)  [unwired: 7 in]
        n499 = case shown="True" w913 {
          selector: w913 -> [_ w928]
          frame False {
          }
          frame True {
            n500 = property on="Confirm 3rd Point" class="Bool (strict)"("Val(Sgnl)"=w928) -> ()  [unwired: 2 in, 2 out]
          }
        }
        n501 = Bundle By Name(cluster=w917, "DMM Connected"=w918, "Output Reading"=w913) -> (w916:T7)
        n502 = Insert Into Array(array=w924, index=0, new element=string[] ["Main", "Final Cal Point"]) -> (w925:string[])
      }
      frame "Calculate Coeffs" {
        w931 = 1000.0 ("Cal Value 3")
        w939 = T9."Enabled" ("Disabled")
        w945 = T9."Disabled and Grayed Out" ("Disabled")
        n503 = local read "Reading Value 1"() -> (w962:dbl)
        n504 = local read "Reading Value 2"() -> (w961:dbl)
        n505 = local read "Reading Value 3"() -> (w960:dbl)
        n506 = Unbundle By Name(w949) -> ("Cal Unit"=w937:T3, "Verification"=w938:bool, "Netway"=w956:i32, "Channel to Cal"=w955:T2, "In/Out"=w946:T1)
        n507 = Build Array("Cal Value 1", "Cal Value 2", "Cal Value 3") -> (w933:dbl[])
        n508 = Build Array(w962, w961, w960) -> (w932:dbl[])
        n509 = Multiply(x=w933, y=w931) -> (x*y=w930:dbl[])
        n510 = Multiply(x=w932, y=w931) -> (x*y=w929:dbl[])
        n511 = property on="Reading Value 3" class="DigNum (strict)"("DisabledEnum"=w945) -> ()  [unwired: 2 in, 2 out]
        n512 = property on="Cal Value 3" class="DigNum (strict)"("DisabledEnum"=w945) -> ()  [unwired: 2 in, 2 out]
        n513 = property on="Confirm 3rd Point" class="Bool (strict)"("DisabledEnum"=w945) -> ()  [unwired: 2 in, 2 out]
        n514 = property on="Cal Table" class="Tbl (strict)"("DisabledEnum"=w945) -> ()  [unwired: 2 in, 2 out]
        n515 = property on="Save Cal" class="Bool"("DisabledEnum"=T9."Enabled" ("Disabled")) -> ()  [unwired: 2 in, 2 out]
        n516 = call <vilib>:"General Polynomial Fit Coefficients.vi"("Y"=w930, "polynomial order"=2, "X"=w929) -> ("Polynomial Coefficients"=w959:dbl[])  [unwired: 11 in, 1 out]
        n517 = Index Array(array=w959) -> (element #1=w936:dbl, element #2=w935:dbl, element #3=w934:dbl)  [unwired: 3 in]
        n518 = case shown="True" w938 {
          tunnel: w956 -> [w986 _]
          tunnel: w955 -> [w985 _]
          tunnel: [w984 errorcluster {"status"=FALSE, "code"=0, "source"=""} ("Error OUT")] -> w947
          tunnel: w946 -> [w983 _]
          tunnel: w936 -> [w981 _]
          tunnel: w935 -> [w980 _]
          tunnel: w934 -> [w979 _]
          frame False {
            n519 = call "Write Cal Parameters.vi"("Serial Number"=w986, "Store (T)"=FALSE, "a0"=w981, "a1"=w980, "a2"=w979, "Channel"=w985, "In/Out"=w983) -> ("Error OUT"=w984:errorcluster)  [unwired: 8 in]
          }
          frame True {
          }
        }
        n520 = property on="Verify Tab" class="TabCtl (strict)"("Visible"=TRUE) -> (error out=w941:errorcluster)  [unwired: 2 in, 1 out]
        n521 = property on="f(x)" class="DigNum (strict)"("DisabledEnum"=w939) -> ()  [unwired: 2 in, 2 out]
        n522 = property on="a0" class="DigNum (strict)"("DisabledEnum"=w939) -> ()  [unwired: 2 in, 2 out]
        n523 = property on="a1" class="DigNum (strict)"("DisabledEnum"=w939) -> ()  [unwired: 2 in, 2 out]
        n524 = property on="a2" class="DigNum (strict)"("DisabledEnum"=w939) -> ()  [unwired: 2 in, 2 out]
        n525 = case shown="\"V\", Default" w937 {
          tunnel: w956 -> [w976 _]
          tunnel: w955 -> [w975 _]
          tunnel: [w974 w977] -> w954
          tunnel: [w973 w977] -> w953
          tunnel: [w972 w977] -> w952
          tunnel: [w971 w978] -> w951
          tunnel: w947 -> [w970 w978]
          tunnel: w946 -> [w969 _]
          frame "V", Default {
            n526 = call "Read Cal Parameters.vi"("Error IN"=w970, "In/Out"=w969, "Channel"=w975, "Serial Number"=w976) -> ("Error OUT"=w971:errorcluster, "a2"=w972:dbl, "a1"=w973:dbl, "a0"=w974:dbl)  [unwired: 4 in]
          }
          frame "%", "Hz" {
            w977 = 0.0 ("a0")
          }
        }
        "a0" <- w954
        "a2" <- w952
        "a1" <- w953
        n527 = property on="Verify Table" class="Tbl (strict)"(error in=w941, "Key Focus"=TRUE, "EditPos"=T10 {"Row"=0, "Column"=1} ("Active Cell:Active Cell")) -> ()  [unwired: 1 in, 2 out]
        n528 = Merge Errors(w951, w947) -> (w950:errorcluster)
        n529 = case shown="No Error" w950 {
          tunnel: [w993 string[] ["End Cal"]] -> w968
          tunnel: w949 -> [w992 w996]
          tunnel: [w991 w996] -> w948
          tunnel: w946 -> [w988 _]
          frame No Error {
            n530 = case shown="\"Input\", Default" w988 {
              tunnel: [string[] ["Cal Review"] string[] ["Set Output", "Cal Review"]] -> w993
              frame "Input", Default {
              }
              frame "Output" {
              }
            }
            n531 = Bundle By Name(cluster=w992, "Output Index"=u8 0, "Review"=TRUE) -> (w991:T7)
          }
          frame Error {
            n532 = One Button Dialog(message="Failed to write cal coefficients to Netway.  Calibration of this channel will now be terminated.") -> ()  [unwired: 1 in, 1 out]
          }
        }
        n533 = Insert Into Array(array=w966, index=0, new element=w968) -> (w967:string[])
      }
      frame "Cal Review" {
        n534 = Unbundle By Name(w1015) -> ("Init Mean"=w1007:bool, "Netway"=w1012:i32, "Channel to Cal"=w1011:T2, "Cal Unit"=w1010:T3, "In/Out"=w1009:T1, "DMM Connected"=w1008:bool, "Auto"=w1020:bool, "Verify Table"=w1019:string[][])
        n535 = property on="Verify Table" class="Tbl (strict)"() -> ("EditPos"=w1013:T10)  [unwired: 2 in, 2 out]
        n536 = Unbundle(w1013) -> ("Row"=w1036:i32)  [unwired: 1 out]
        n537 = Greater Or Equal To 0?(x=w1036) -> (x >= 0?=w1037:bool)
        n538 = Index Array(array=w1019, index (row)=w1036, index (col)=0 ("disabled index (col)")) -> (element=w1029:string)
        n539 = Fract/Exp String To Number(string=w1029) -> (number=w1032:dbl)  [unwired: 3 in, 1 out]
        n540 = case shown="False" w1037 {
          tunnel: w1036 -> [_ w1039]
          frame False {
          }
          frame True {
            "Row" <- w1039
          }
        }
        n541 = Increment(x=w1032) -> (x+1=w1031:dbl)
        n542 = local read "avg"() -> (w1005:i32)
        n543 = Empty String/Path?(string/path=w1029) -> (empty?=w1028:bool)
        n544 = Not(x=w1028) -> (.not. x?=w1001:bool)
        n545 = call "Get Cal Point.vi"("Netway"=w1012, "Init Mean"=w1007, "Channel to Cal"=w1011, "Cal Unit"=w1010, "In/Out"=w1009, "DMM Connected in"=w1008, "avg"=w1005) -> ("DMM Connected out"=w1006:bool, "Output Reading"=w1000:bool, "Reading"=w1004:dbl)  [unwired: 6 in]
        "f(x)" <- w1004
        n546 = Increment(x=w1004) -> (x+1=w1030:dbl)
        n547 = Subtract(x=w1030, y=w1031) -> (x-y=w1018:dbl)
        n548 = Divide(x=w1018, y=w1030) -> (x/y=w1017:dbl)
        n549 = Absolute Value(x=w1017) -> (abs(x)=w1016:dbl)
        n550 = Less?(x=w1016, y=0.1) -> (x < y?=w1033:bool)
        n551 = Compound Arithmetic op=AND(w1020, w1033, w1001) -> (w1027:bool)
        n552 = And(x=w1000, y=w1001) -> (x .and. y?=w999:bool)
        n553 = call "Reading Delay.vi"("Delay"="ms", "In Range"=w1027) -> ("Take Reading"=w1003:bool)  [unwired: 9 in]
        n554 = Or(x=w999, y=w1003) -> (x .or. y?=w1002:bool)
        n555 = case shown="True" w1002 {
          selector: w1002 -> [_ w1038]
          frame False {
          }
          frame True {
            n556 = property on="Verify Read" class="Bool (strict)"("Val(Sgnl)"=w1038) -> ()  [unwired: 2 in, 2 out]
          }
        }
        n557 = Insert Into Array(array=w1023, index=0, new element=string[] ["Main", "Cal Review"]) -> (w1024:string[])
        n558 = Bundle By Name(cluster=w1015, "Init Mean"=FALSE, "DMM Connected"=w1006, "Output Reading"=w1000) -> (w1021:T7)
      }
      frame "Save Cal" {
        n559 = Unbundle By Name(w1047) -> ("Cal Unit"=w1046:T3, "Channel to Cal"=w1045:T2, "In/Out"=w1042:T1, "Netway"=w1044:i32, "Channel to Cal"=w1043:T2, "Verification"=w1040:bool)
        n560 = case shown="False" w1040 {
          tunnel: w1046 -> [w1062 _]
          tunnel: w1045 -> [w1061 _]
          tunnel: w1042 -> [w1060 _]
          frame False {
            n561 = case shown="\"V\"" w1062 {
              tunnel: w1061 -> [_ w1063]
              tunnel: w1060 -> [_ w1065]
              frame Default {
              }
              frame "V" {
                w1073 = u16 4 ("y")
                n562 = case shown="\"Output\"" w1065 {
                  tunnel: [w1078 w1079] -> w1064
                  tunnel: w1063 -> [w1078 w1081]
                  frame "Input", Default {
                  }
                  frame "Output" {
                    n563 = Add(x=w1081, y=8) -> (x+y=w1079:i32)
                  }
                }
                n564 = Bundle(cluster=T10 {"Row"=0, "Column"=0} ("Active Cell:Active Cell"), "Row"=w1064, "Column"=-2) -> (w1074:T10)
                n565 = Greater?(x=w1064, y=w1073) -> (0:w1072:bool)
                n566 = Subtract(x=w1064, y=w1073) -> (x-y=w1071:i32)
                n567 = Select(t=w1071, s=w1072, f=u16 0 ("y")) -> (s? t:f=w1068:i32)
                n568 = Bundle(cluster=T10 {"Row"=0, "Column"=0} ("Active Cell:Active Cell"), "Row"=w1068, "Column"=0) -> (w1067:T10)
                n569 = property on="Cal Table" class="Tbl (strict)"("Active Cell"=w1074, "Cell BG Color"=u32 16775793, "Index Values"=w1067) -> ()  [unwired: 2 in, 2 out]
              }
            }
          }
          frame True {
          }
        }
        n570 = case shown="False" w1040 {
          tunnel: w1044 -> [w1058 _]
          tunnel: w1043 -> [w1054 _]
          tunnel: w1042 -> [w1053 _]
          tunnel: [w1052 errorcluster {"status"=FALSE, "code"=0, "source"=""} ("Error OUT")] -> w1041
          frame False {
            n571 = local read "a0"() -> (w1057:dbl)
            n572 = local read "a1"() -> (w1056:dbl)
            n573 = local read "a2"() -> (w1055:dbl)
            n574 = call "Write Cal Parameters.vi"("Serial Number"=w1058, "a0"=w1057, "a1"=w1056, "a2"=w1055, "Channel"=w1054, "In/Out"=w1053) -> ("Error OUT"=w1052:errorcluster)  [unwired: 9 in]
          }
          frame True {
          }
        }
        n575 = case shown="No Error" w1041 {
          tunnel: [string[] ["Load Coefficients", "Write to Excel", "Increment Channel", "End Cal"] string[] ["End Cal"]] -> w1048
          frame No Error {
          }
          frame Error {
            n576 = One Button Dialog(message="Failed to save coefficients to non-volatile memory on Netway.  Calibration of this channel will now be terminated.") -> ()  [unwired: 1 in, 1 out]
          }
        }
        n577 = Insert Into Array(array=w1050, index=0, new element=w1048) -> (w1051:string[])
      }
      frame "Calc Dev" {
        n578 = Unbundle By Name(w1089) -> ("Verify Table"=w1092:string[][], "Cal Unit"=w1095:T3, "Channel to Cal"=w1085:T2, "Verify Table Ref"=w1093:refnum<vi>)
        n579 = call "Calc Dev (Netway).vi"("Verify Table IN"=w1092, "Units"=w1095, "Channel to Cal"=w1085, "Dev Table 1 Ref"=w1093) -> ("Verify Table OUT"=w1094:string[][])  [unwired: 15 in]
        n580 = local write "Verify Table"(w1094) -> ()
        n581 = Bundle By Name(cluster=w1089, "Verify Table"=w1094) -> (w1088:T7)
        n582 = Insert Into Array(array=w1086, index=0, new element=string[] []) -> (w1087:string[])
      }
      frame "Write to Excel" {
        n583 = Unbundle By Name(w1102) -> ("Cal Spreadsheet Path"=w1103:path, "Verify Table"=w1106:string[][], "Channel to Cal"=w1107:T2, "Cal Unit"=w1108:T3, "In/Out"=w1098:T1, "ZGW?"=w1096:bool)
        n584 = flat-sequence {
          tunnel: w1103 -> [w1120]
          tunnel: [w1120] -> w1112
          tunnel: [w1117] -> w1111
          tunnel: w1106 -> [w1117]
          tunnel: [w1116] -> w1110
          tunnel: w1107 -> [w1116]
          tunnel: [w1115] -> w1109
          tunnel: w1108 -> [w1115]
          tunnel: [w1114] -> w1099
          tunnel: w1098 -> [w1114]
          tunnel: [w1113] -> w1097
          tunnel: w1096 -> [w1113]
          tunnel: w1112 -> [w1126]
          tunnel: w1111 -> [w1125]
          tunnel: w1110 -> [w1124]
          tunnel: w1109 -> [w1123]
          tunnel: w1099 -> [w1122]
          tunnel: w1097 -> [w1121]
          frame #0 {
            n585 = property on="Main Tab" class="TabCtl (strict)"("DisabledEnum"=T9."Disabled" ("Disabled")) -> ()  [unwired: 2 in, 2 out]
            n586 = property on="Load Indicator Tab" class="TabCtl (strict)"("Visible"=TRUE) -> ()  [unwired: 2 in, 2 out]
          }
          frame #1 {
            n587 = call "Write Netway Data.vi"("ZGW?"=w1121, "In/Out"=w1122, "Cal Unit"=w1123, "Channel"=w1124, "Verify Table"=w1125, "Cal Path"=w1126) -> ()  [unwired: 6 in]
          }
          frame #2 {
            n588 = property on="Main Tab" class="TabCtl (strict)"("DisabledEnum"=T9."Enabled" ("Disabled")) -> ()  [unwired: 2 in, 2 out]
            n589 = property on="Load Indicator Tab" class="TabCtl (strict)"("Visible"=FALSE) -> ()  [unwired: 2 in, 2 out]
          }
        }
        n590 = Insert Into Array(array=w1101, index=0, new element=string[] ["Recolor Tables"]) -> (w1100:string[])
      }
      frame "Recolor Tables" {
        n591 = Unbundle By Name(w1130) -> ("Verify Table Ref"=w1133:refnum<vi>)
        n592 = property on="Property Node" class="Tbl (strict)"(reference=w1133, "Active Cell"=T10 {"Row"=-2, "Column"=-2} ("Active Cell:Active Cell"), "Cell BG Color"=u32 15527148) -> (reference out=w1136:refnum<vi>)  [unwired: 1 in, 1 out]
        n593 = property on="Property Node" class="Tbl (strict)"(reference=w1136, "Active Cell"=T10 {"Row"=-2, "Column"=1} ("Active Cell:Active Cell"), "Cell BG Color"=u32 16448250) -> ()  [unwired: 1 in, 2 out]
      }
      frame "End Cal" {
        w1146 = FALSE ("Visible")
        w1145 = T9."Enabled" ("Disabled")
        w1147 = T9."Disabled and Grayed Out" ("Disabled")
        w1137 = 0.0 ("Cal Value 1")
        n594 = Unbundle By Name(w1138) -> ("Cal Spreadsheet Path"=w1144:path)
        n595 = property on="Header" class="Bool"("DisabledEnum"=w1145) -> ()  [unwired: 2 in, 2 out]
        n596 = property on="Main Tab" class="TabCtl (strict)"("DisabledEnum"=w1145) -> ()  [unwired: 2 in, 2 out]
        n597 = Empty String/Path?(string/path=w1144) -> (empty?=w1140:bool)
        n598 = Select(t=2, s=w1140, f=0) -> (s? t:f=w1139:i32)
        n599 = property on="Header OK" class="Bool"("DisabledEnum"=w1147) -> ()  [unwired: 2 in, 2 out]
        n600 = property on="Header Cancel" class="Bool"("DisabledEnum"=w1147) -> ()  [unwired: 2 in, 2 out]
        n601 = property on="Netway" class="DigNum (strict)"("DisabledEnum"=w1139) -> ()  [unwired: 2 in, 2 out]
        n602 = property on="Channel to Cal" class="Enum (strict)"("DisabledEnum"=w1139) -> ()  [unwired: 2 in, 2 out]
        n603 = property on="Start Cal" class="Bool"("DisabledEnum"=w1139) -> ()  [unwired: 2 in, 2 out]
        n604 = property on="Cal Unit" class="Enum (strict)"("DisabledEnum"=w1139) -> ()  [unwired: 2 in, 2 out]
        n605 = property on="Start Verification" class="Bool"("DisabledEnum"=w1139) -> ()  [unwired: 2 in, 2 out]
        n606 = property on="View Spreadsheet" class="Bool"("DisabledEnum"=w1139) -> ()  [unwired: 2 in, 2 out]
        n607 = property on="In/Out" class="Enum (strict)"("DisabledEnum"=w1139) -> ()  [unwired: 2 in, 2 out]
        n608 = local write "Cancel Cal"(FALSE ("Cancel Cal")) -> ()
        n609 = property on="Header Tab" class="TabCtl (strict)"("Visible"=w1146) -> ()  [unwired: 2 in, 2 out]
        n610 = property on="Load Indicator Tab" class="TabCtl (strict)"("Visible"=w1146) -> ()  [unwired: 2 in, 2 out]
        n611 = local write "Reading Value 1"(w1137) -> ()
        n612 = local write "Reading Value 2"(w1137) -> ()
        n613 = local write "Reading Value 3"(w1137) -> ()
        n614 = local write "Cal Value 1"(w1137) -> ()
        n615 = local write "Cal Value 2"(w1137) -> ()
        n616 = local write "Cal Value 3"(w1137) -> ()
        n617 = local write "a0"(w1137) -> ()
        n618 = local write "a1"(w1137) -> ()
        n619 = local write "a2"(w1137) -> ()
        n620 = local write "f(x)"(w1137) -> ()
      }
      frame "Increment Channel" {
        n621 = Unbundle By Name(w1151) -> ("Channel to Cal"=w1153:T2)
        n622 = Increment(x=w1153) -> (x+1=w1152:T2)
        n623 = local write "Channel to Cal"(w1152) -> ()
        n624 = Bundle By Name(cluster=w1151, "Channel to Cal"=w1152) -> (w1150:T7)
      }
      frame "Check Firmware" {
        n625 = Unbundle By Name(w1159) -> ("Firmware Version"=w1157:string, "Netway"=w1155:i32)
        n626 = call "Get Firmware Version.vi"("Serial Number"=w1155) -> ("Firmware Version"=w1158:string)  [unwired: 9 in, 1 out]
        n627 = call <vilib>:"Trim Whitespace.vi"("string"=w1158) -> ("trimmed string"=w1156:string)  [unwired: 1 in]
        n628 = call "Check Firmware.vi"("Actual"=w1156, "Cut-off"=w1157) -> ("New Enough?"=w1154:bool)  [unwired: 9 in]
        n629 = case shown="False" w1154 {
          tunnel: [string[] ["End Cal"] w1167] -> w1161
          tunnel: w1160 -> [_ w1167]
          tunnel: w1157 -> [w1163 _]
          tunnel: w1156 -> [w1162 _]
          frame False {
            n630 = Format Into String(format string="Firmware version is too old to properly perform a calibration :(\n\nYour current version is %s\n\nMake sure Netway is at least version %s" ("message"), w1162, w1163) -> (resulting string=w1164:string)  [unwired: 2 in, 1 out]
            n631 = One Button Dialog(message=w1164) -> ()  [unwired: 1 in, 1 out]
          }
          frame True {
          }
        }
      }
      frame "Check Software" {
        n632 = Unbundle By Name(w1173) -> ("Software Version"=w1172:string)
        n633 = call "Get Netway App Version.vi"("Cut-off"=w1172) -> ("New Enough?"=w1169:bool, "Software Installed?"=w1168:bool, "Current Version"=w1171:string)  [unwired: 11 in, 1 out]
        n634 = And(x=w1169, y=w1168) -> (x .and. y?=w1170:bool)
        n635 = case shown="False" w1170 {
          tunnel: [string[] ["End Cal"] w1185] -> w1175
          tunnel: w1174 -> [_ w1185]
          tunnel: w1172 -> [w1178 _]
          tunnel: w1171 -> [w1183 _]
          tunnel: w1168 -> [w1182 _]
          frame False {
            n636 = Format Into String(format string="Netway application version is too old to properly perform a calibration :(\n\nYour current version is %s\n\nMake sure Netway application is at least version %s" ("message"), w1183, w1178) -> (resulting string=w1180:string)  [unwired: 2 in, 1 out]
            n637 = Format Into String(format string="The Netway application is not installed on this computer.\n\nYou must install version %s before running this Cal Utility." ("message"), w1178) -> (resulting string=w1177:string)  [unwired: 2 in, 1 out]
            n638 = Select(t=w1180, s=w1182, f=w1177) -> (s? t:f=w1176:string)
            n639 = One Button Dialog(message=w1176) -> ()  [unwired: 1 in, 1 out]
          }
          frame True {
          }
        }
      }
      frame "Exit" {
        n640 = call "Keithly 2000 Global.vi"("Mode (Read)"=enum16{"Init", "Read DC Volts", "Close"}."Close") -> ("error out"=w1186:errorcluster)  [unwired: 9 in, 1 out]
        n641 = call <vilib>:"Clear Errors.vi"("error in (no error)"=w1186) -> ()  [unwired: 6 in, 1 out]
      }
    }
  }
